vi "OP_Print_TPS_cluster_20170928.vi"() -> ()   [LabVIEW 2013]
uses:
  <vilib>/addons/database/Connection.llb/DB Tools Open Connec (Path).vi
  <vilib>/addons/database/Connection.llb/Conn Execute.vi
  <vilib>/addons/database/Recordset.llb/Rec Fetch Recordset Data (R).vi
  <vilib>/addons/database/Recordset.llb/Rec Destroy - Connection.vi
  <userlib>/caLab/Private/Get_PV-1D.vi
  <userlib>/caLab/Private/Get_PV.vi
  <vilib>/addons/database/NI_Database_API.lvlib
panel:
  in  "Refresh Button":bool
  in  "last ? Hrs":dbl=12.0 min=1.0 max=24.0 step=1.0
  out "error out 2":errorcluster
  out "x = y?":bool
  out "NOW time":string="21:22:35"
  out "NOW date":string="2017/09/13"
  in  "Save Button":bool
  out "error out 3":errorcluster
  in  "stop":bool
  out "time kickeron":string="21:11:02"
  out "date kickeron":string="2017/09/13"
  out "Cluster":T1={"SR Fill Pattern"=array[864 elements], "Beam Current(mA"=301.29559, "Beam Lifetime(min)"=467.3623843429031, "Beamsize X(um)"=61.81771808059018, "Beamsize Y(um)"=34.43346871436747, "Tune X(from BPM)"=0.0, "Tune Y(from BPM)"=0.0, "Mode"="Top-Up", "NuX(from BBF) "=0.15280663925802224, "NuY(from BBF)"=0.22496346361412184, "IU22-23gap(R)"=7.0, "IU22-05gap(R)"=7.28, "IU22-05M"=TRUE, "IU22A-09gap(R)"=8.058, "IU22A-09M"=TRUE, "IU22B-09gap(R)"=40.001, "IU22B-09M"=FALSE, "IUT22-21gap(R)"=7.0, "IUT22-21M"=TRUE, "IU22-23M"=TRUE, "IU22A-25gap(R)"=7.0, "IU22A-25M"=TRUE, "IU22B-25gap(R)"=40.0, "IU22B-25M"=FALSE, "EPU48A-41gap(R)"=65.0, "EPU48A-41gM"=FALSE, "EPU48B-41gap(R)"=44.99995, "EPU48B-41gM"=TRUE, "EPU46-45gap(R)"=65.00120000000001, "EPU46-45gM"=FALSE, "EPU48A-41phase(R)"=0.0009500000000000001, "EPU48B-41phase(R)"=0.0, "EPU46-45phase(R)"=0.0, "Grid volt.(V)(S)"=33.0, "Gun mode"="MBM", "Mod.3 HV(kV)(S)"=35.519999999999996, "SR"="SR_DMB_2017_0910_1700LOCO.data", "BR"="Booster_JT_2017_0714_1140.data", "Linac"="Linac_2017_0413_1015.data", "LTB"="LTB_JT_2017_0828_1050.data", "BTS"="BTS_2017_0911_0610.data", "RF2 remote"=TRUE, "RF2 OP mode"=TRUE, "RF2 phase.(S)"=-36.2, "RF Freq.(s)"=499655122.5507494, "RF2 gap volt.(S)"=1400.0, "RF3 remote"=TRUE, "RF3 OP mode"=TRUE, "RF3 phase.(S)"=9.000000000000004, "RF3 gap volt.(S)"=1400.0, "BBF V"=TRUE, "BBF H"=TRUE, "BR ext. kicker1(kV)"=17.666, "BR ext. kicker2(kV)"=17.666, "BR ext. sep.1(V)"=322.14, "BR ext. sep.2(V)"=441.1, "BR inj. sep.(V)"=104.95, "BR inj. kicker(kV)"=12.131749999999993, "SR kicker4(kV)"=8.133, "SR kicker3(kV)"=7.798, "SR kicker2(kV)"=8.259, "SR kicker1(kV)"=8.2, "SR inj. sep.2(V)"=397.2, "SR inj. sep.1(V)"=398.04, "Bucket Start"=100.0, "Bucket Last"=600.0, "Bucket Step"=10.0, "Orbit ILK(P)"=TRUE, "IU22-05 Hutch Enable"=TRUE, "IU22A-09M Hutch Enable"=TRUE, "IUT22-21M Hutch Enable"=TRUE, "IU22-23M Hutch Enable"=TRUE, "IU22A-25M Hutch Enable"=TRUE, "EPU48A-41M Hutch Enable"=FALSE, "EPU46-45M Hutch Enable"=FALSE, "EPU46-45 FE Enable"=TRUE, "EPU48A-41 FE Enable"=TRUE, "IU22A-25 FE Enable"=TRUE, "IU22-23 FE Enable"=TRUE, "IUT22-21 FE Enable"=TRUE, "IU22A-09 FE Enable"=TRUE, "IU22-05 FE Enable"=TRUE, "EPU48A-41pM"=FALSE, "EPU48B-41pM"=TRUE, "EPU46-45pM"=FALSE, "Gun volt.(V)(S)"=23.5, "Width count"=30.0, "2ns step"=0.0, "10ps delay"=150.0, "phase shifter"=130.0021, "Taper"=1.0899999999999999, "05XBPMX 1"=-12.071, "09XBPMX 1"=236.232, "21XBPMX 1"=109.949, "23XBPMX 1"=-54.123000000000005, "25XBPMX 1"=836.426, "41XBPMX 1"=-393.619, "45XBPMX 1"=-542.557, "05XBPMY 1"=49.623, "09XBPMY 1"=-49.685, "21XBPMY 1"=1810.249, "23XBPMY 1"=8.221, "25XBPMY 1"=-161.43800000000002, "41XBPMY 1"=188.45000000000002, "45XBPMY 1"=-785.827, "FOFB H"="On", "FOFB V"="On", "time string"="21:22:35", "date"="2017/09/13", "date (last kicker ON)"="2017/09/13", "time string (last kicker ON)"="21:11:02", "BPMX Graph"={[1, 2, 3, 4, 5, 6, 7, 8, 9, 10, 11, 12, 13, 14, 15, 16, 17, 18, 19, 20, 21, 22, 23, 24, 25, 26, 27, 28, 29, 30, 31, 32, 33, 34, 35, 36, 37, 38, 39, 40, 41, 42, 43, 44, 45, 46, 47, 48, 49, 50, 51, 52, 53, 54, 55, 56, 57, 58, 59, 60, 61, 62, 63, 64, 65, 66, 67, 68, 69, 70, 71, 72, 73, 74, 75, 76, 77, 78, 79, 80, 81, 82, 83, 84, 85, 86, 87, 88, 89, 90, 91, 92, 93, 94, 95, 96, 97, 98, 99, 100, 101, 102, 103, 104, 105, 106, 107, 108, 109, 110, 111, 112, 113, 114, 115, 116, 117, 118, 119, 120, 121, 122, 123, 124, 125, 126, 127, 128, 129, 130, 131, 132, 133, 134, 135, 136, 137, 138, 139, 140, 141, 142, 143, 144, 145, 146, 147, 148, 149, 150, 151, 152, 153, 154, 155, 156, 157, 158, 159, 160, 161, 162, 163, 164, 165, 166, 167, 168, 169, 170, 171, 172, 173, 174], "1rst Value (number)"=[-57.953, -16.830000000000002, -69.81400000000001, 33.217, 55.747, -102.116, 112.23700000000001, -53.109, -8.106, -108.797, 42.098, -26.618000000000002, 23.191, -14.290000000000001, -1.155, -135.518, -122.34, 81.94200000000001, -31.955000000000002, -107.23100000000001, 144.648, -41.501, -20.927, -71.483, 72.117, 174.239, 163.291, 218.172, -123.111, -19.648, 721.419, 453.44, -205.66400000000002, 29.594, 134.439, -81.831, 78.56700000000001, 81.661, 6.593, -174.97, 3.722, 159.74, -88.646, 74.924, 15.269, -34.265, -113.105, -24.846, 66.414, -131.589, 93.44500000000001, 99.491, -12.985, -180.05100000000002, 131.165, 37.079, -154.526, 160.38400000000001, 49.599000000000004, 24.96, -73.793, 85.367, 37.467, -10.198, 89.935, -39.093, 45.050000000000004, -60.443, 91.7, -89.60600000000001, -338.463, -13.786, -319.98900000000003, -247.719, -134.31, 117.925, -10.984, -69.336, 71.378, -119.991, 35.43, -76.868, 56.546, -1.875, -582.236, -130.956, -298.747, -39.141, 76.82900000000001, 82.033, -47.447, 68.075, 11.526, -161.376, 200.095, -3.3000000000000003, -170.391, -174.619, -59.896, 50.463, -167.593, 164.144, 6.708, -52.142, -152.178, 67.056, 8.861, -173.928, 197.31, 48.799, -71.952, -62.230000000000004, -4.128, 137.421, -127.104, 79.596, 56.283, -67.373, -122.31400000000001, 36.139, 42.783, -82.897, 55.373000000000005, 14.632, -53.128, -78.393, 32.919000000000004, -27.649, -194.787, 148.28300000000002, 205.038, -156.17600000000002, -87.652, -24.492, 101.044, -122.638, 98.552, 5.809, 62.325, -64.294, 38.297000000000004, 46.068, 274.628, 436.098, -130.642, -298.747, 133.037, 11.423, -153.334, 114.726, 76.023, -90.009, 92.394, 59.627, -74.368, -118.376, 43.591, 66.153, -129.306, 168.713, 4.539, -35.064, -130.217, 42.444, 59.192, -125.98400000000001, 147.53, 66.584, -28.801000000000002, -176.53, 75.164, 77.199, -57.284, -9.878]}, "BPMY Graph"={[1, 2, 3, 4, 5, 6, 7, 8, 9, 10, 11, 12, 13, 14, 15, 16, 17, 18, 19, 20, 21, 22, 23, 24, 25, 26, 27, 28, 29, 30, 31, 32, 33, 34, 35, 36, 37, 38, 39, 40, 41, 42, 43, 44, 45, 46, 47, 48, 49, 50, 51, 52, 53, 54, 55, 56, 57, 58, 59, 60, 61, 62, 63, 64, 65, 66, 67, 68, 69, 70, 71, 72, 73, 74, 75, 76, 77, 78, 79, 80, 81, 82, 83, 84, 85, 86, 87, 88, 89, 90, 91, 92, 93, 94, 95, 96, 97, 98, 99, 100, 101, 102, 103, 104, 105, 106, 107, 108, 109, 110, 111, 112, 113, 114, 115, 116, 117, 118, 119, 120, 121, 122, 123, 124, 125, 126, 127, 128, 129, 130, 131, 132, 133, 134, 135, 136, 137, 138, 139, 140, 141, 142, 143, 144, 145, 146, 147, 148, 149, 150, 151, 152, 153, 154, 155, 156, 157, 158, 159, 160, 161, 162, 163, 164, 165, 166, 167, 168, 169, 170, 171, 172, 173, 174], "1rst Value (number)"=[-151.316, -17.054000000000002, -19.178, 120.799, -59.688, 21.818, 7.809, -29.198, 24.311, 16.134, -40.005, -27.325, 53.925000000000004, 3.1670000000000003, -9.254, 61.293, -34.105000000000004, 94.741, -29.063, -23.54, 22.793, 14.087, -38.574, 36.56, -99.245, -0.044, 48.661, 33.093, -212.454, -68.398, 390.704, 121.525, -58.935, -19.379, 2.579, -18.495, 19.617, -37.129, 48.386, 12.363, -36.386, 3.988, 67.735, -11.383000000000001, 4.172, -13.203, 10.164, -0.589, -22.969, 30.752, -38.915, 41.105000000000004, -21.456, -4.901, 29.631, -9.992, -32.032000000000004, 12.132, -68.125, 97.674, -58.86, 66.602, -68.949, 58.512, -42.012, 22.742, -15.959, 12.297, 5.471, -82.755, 65.11, 15.540000000000001, -166.881, -18.198, 7.187, -10.503, 30.153000000000002, -70.941, -3.086, 7.163, -7.828, -18.855, 26.188, -7.574, 38.271, 0.135, -13.549, 40.546, 139.87800000000001, 4.58, -2.962, -6.871, 5.808, 0.435, 13.713000000000001, -7.65, -7.087, -2.88, 14.262, -32.895, 32.566, -5.7620000000000005, -44.698, 76.731, -22.138, 22.336000000000002, -6.075, -10.424, 12.001, -9.495000000000001, 18.714, -1.697, 7.412, -43.832, 47.095, -41.426, 2.965, 43.068, 29.560000000000002, -31.904, 28.699, -0.466, -7.138, -5.288, -15.559000000000001, 34.502, -45.603, -18.644000000000002, -3.043, -37.238, -6.869, -15.336, -4.0600000000000005, 13.134, -43.802, 53.087, -14.268, -32.236000000000004, 35.516, -16.788, 25.02, -56.714, 59.035000000000004, 117.801, 64.776, -29.192, -39.944, 137.099, -65.81700000000001, 24.237000000000002, -41.801, 16.21, 15.972, -22.743000000000002, 31.377, 18.596, 7.515000000000001, -19.796, 10.161, 1.0070000000000001, -7.114, -12.046, -4.223, 21.048000000000002, -8.239, -20.592, -8.097, 90.321, -136.733, 37.556, 84.604, -63.991, 30.307000000000002, 1.127]}, "Radio Buttons 2"=enum."absolute", "09XBPMX 2"="-47.22", "09XBPMY 2"="-3.76", "05XBPMY 2"="-491.14", "05XBPMX 2"="-472.70", "21XBPMY 2"=" closed", "21XBPMX 2"=" PAB ", "23XBPMY 2"="188.03", "23XBPMX 2"="-8.61", "25XBPMY 2"="5165.53", "25XBPMX 2"="2146.38", "41XBPMY 2"=" closed", "41XBPMX 2"=" Hutch ", "45XBPMX 2"=" Hutch ", "45XBPMY 2"=" closed", "05 mode"="Follow", "09A mode"="Follow", "09B mode"="Follow", "21 mode"="Follow", "23 mode"="Follow", "25A mode"="Follow", "25B mode"="Follow", "41A mode"="Follow", "41B mode"="Follow", "46 mode"="Follow", "BeamCurrent History"={"BPM NO.  1_172"=array[4320 elements], array[4320 elements]}, "SR Beam Current in            hours"=12.0} {"SR Beam Current in            hours" min=1.0 max=24.0 step=1.0 format="%#_2f"; "45XBPMY 1" format="%#.2f"; "41XBPMY 1" format="%#.2f"; "25XBPMY 1" format="%#.2f"; "23XBPMY 1" format="%#.2f"; "21XBPMY 1" format="%#.2f"; "09XBPMY 1" format="%#.2f"; "05XBPMY 1" format="%#.2f"; "45XBPMX 1" format="%#.2f"; "41XBPMX 1" format="%#.2f"; "25XBPMX 1" format="%#.2f"; "23XBPMX 1" format="%#.2f"; "21XBPMX 1" format="%#.2f"; "09XBPMX 1" format="%#.2f"; "05XBPMX 1" format="%#.2f"; "Taper" format="%#.4f"; "phase shifter" format="%#.3f"; "10ps delay" format="%#.1f"; "2ns step" format="%#.1f"; "Width count" format="%#.1f"; "Gun volt.(V)(S)" format="%#.1f"; "Bucket Step" format="%#.2f"; "Bucket Last" format="%#.2f"; "Bucket Start" format="%#.2f"; "BR ext. kicker1(kV)" format="%#.2f"; "BR ext. kicker2(kV)" format="%#.2f"; "BR ext. sep.1(V)" format="%#.2f"; "BR ext. sep.2(V)" format="%#.2f"; "BR inj. sep.(V)" format="%#.3f"; "BR inj. kicker(kV)" format="%#.3f"; "SR kicker4(kV)" format="%#.2f"; "SR kicker3(kV)" format="%#.2f"; "SR kicker2(kV)" format="%#.2f"; "SR kicker1(kV)" format="%#.2f"; "SR inj. sep.2(V)" format="%#.2f"; "SR inj. sep.1(V)" format="%#.2f"; "RF3 gap volt.(S)" format="%#.0f"; "RF3 phase.(S)" format="%#.1f"; "RF2 gap volt.(S)" format="%#.0f"; "RF Freq.(s)" format="%#.1f"; "RF2 phase.(S)" format="%#.1f"; "Mod.3 HV(kV)(S)" format="%#.3f"; "Grid volt.(V)(S)" format="%#.1f"; "EPU46-45phase(R)" format="%#.4f"; "EPU48B-41phase(R)" format="%#.4f"; "EPU48A-41phase(R)" format="%#.4f"; "EPU46-45gap(R)" format="%#.4f"; "EPU48B-41gap(R)" format="%#.4f"; "EPU48A-41gap(R)" format="%#.4f"; "IU22B-25gap(R)" format="%#.4f"; "IU22A-25gap(R)" format="%#.4f"; "IUT22-21gap(R)" format="%#.4f"; "IU22B-09gap(R)" format="%#.4f"; "IU22A-09gap(R)" format="%#.4f"; "IU22-05gap(R)" format="%#.4f"; "IU22-23gap(R)" format="%#.4f"; "NuY(from BBF)" format="%#.4f"; "NuX(from BBF)" format="%#.4f"; "Tune Y(from BPM)" format="%#.4f"; "Tune X(from BPM)" format="%#.4f"; "Beamsize Y(um)" format="%#.2f"; "Beamsize X(um)" format="%#.2f"; "Beam Lifetime(min)" format="%#.3f"; "Beam Current(mA" format="%#.3f"}
  out "date (last Gun ON)":string="2016/08/29"
  out "time string (last Gun ON)":string="23:28:50"
  out "Value Array (number) 7":dbl[](array[numeric])=[-12.071, 49.623, 236.232, -49.685, 109.949, 1810.249, -54.123000000000005, 8.221, 836.426, -161.43800000000002, -393.619, 188.45000000000002, -542.557, -785.827, -472.696, -491.142, -47.215, -3.761, 16.193, -29.476, -8.605, 188.026, 2146.382, 5165.525000000001, -28.331, 10.717, 132.828, -84.862]
  out "Value Array (number) 6":dbl[](array[numeric])=[7.28, 8.058, 40.001, 7.0, 7.0, 7.0, 40.0, 65.0, 0.0009500000000000001, 44.99995, 0.0, 65.00120000000001, 0.0, -1.0899999999999999, 130.0021]
  out "1rst Value (string) 2":string[](array[string])=["MBM", "33", "23.5", "350", "35.52", "22485", "22485", "62", "30", "0", "0", "200", "150"]
  out "Value Array (number) 5":dbl[](array[numeric])=[499654641.19275105, 1.0, 0.0, 1335.005102558433, 1400.0, -56.1, 1.0, 0.0, 1362.1066276040413, 1400.0, 160.0]
  out "1rst Value (string)":string[](array[string])=["Linac_2017_0413_1015.data", "LTB_JT_2017_0828_1050.data", "Booster_JT_2017_0714_1140.data", "BTS_2017_0911_0610.data", "SR_DMB_2017_0910_1700LOCO.data"]
  out "Value Array (number) 4":dbl[](array[numeric])=[499655122.5507494, 1.0, 0.0, 1326.2153542928932, 1400.0, -36.2, 1.0, 0.0, 1398.366426317367, 1400.0, 9.000000000000004]
  out "Value Array (number) 3":dbl[](array[numeric])=[0.0, 33.0, 23.5, 350.0, 35.519999999999996, 22485.0, 22485.0, 62.0, 30.0, 0.0, 0.0, 200.0, 150.0]
  out "Value Array (number) 2":dbl[](array[numeric])=[104.95, 12.131749999999993, 17.666, 17.666, 322.14, 441.1, 398.04, 397.2, 8.2, 8.259, 7.798, 8.133]
  out "Value Array (number)":dbl[](array[numeric])=[1.0, 301.29559, 467.3623843429031, 51.42904998385207, 28.64681257434898, 0.1761252446183953, 0.12524461839530332, 88.36853790283203, 130.0970458984375, 100.0, 600.0, 10.0]
  out "Orbit ILK(A)":bool
  out "Orbit INT. Ang Active":bool
  out "Orbit INT.Ang. On":bool
  out "Orbit INT. Pos Active":bool
  out "Orbit INT.Pos. On":bool
  out "SBM volt.(S)":dbl=350.0 format="%#.1f"
  out "MBM volt.(S)":dbl=23.5 format="%#.1f"
  in  "Copy Button":bool
  in  "Print Button":bool
  in  "Help Button":bool
  in  "Refresh Button":bool
  in  "Open Button":bool
  out "Gun WCM":dbl[](graph)
  out "BR Fill Pattern":dbl[](graph)
  # "TPS OP Handover Information"
  # "Others"
  # "Time："
  # "Valve  Status"
  # "follow"
  # "SM Status"
  # "歷史電流圖\ntrip次數?\n輻射劑量?\n平均氣壓\n目前最高累計劑量\n最近一次觸發時BR電流及WCM數值"
  # "TPS Operational Handover Information v1.4.1"
  # "SR Status"
  # "Feedback"
  # "Pulse Mag"
  # "LINAC"
  # "x8(ns)"
  # "x2(ns)"
  # "x0.01(ns)"
  # "RF Status"
  # "Hz"
  # "(kV)"
  # "(kV)"
  # "Changeliang@LOP.NSRRC"
  # "SR Fill Pattern"
  # "Lattice Files in using"
  # "ID &Beamline (R)"
  # "mode"
  # "Gap\nmm"
  # "Motor"
  # "Phase"
  # "FE/Hutch"
  # "phase\nshifter"
  # "Taper\n(enc)"
  # "XBPM1X\num"
  # "XBPM1Y\num"
  # "XBPM2X\num"
  # "XBPM2Y\num"
  # "05"
  # "09"
  # "21"
  # "23"
  # "25"
  # "41"
  # "45"
  # "SR Orbit"
  # "BPMX"
  # "BPMY"
  # "SR Beam Current History"
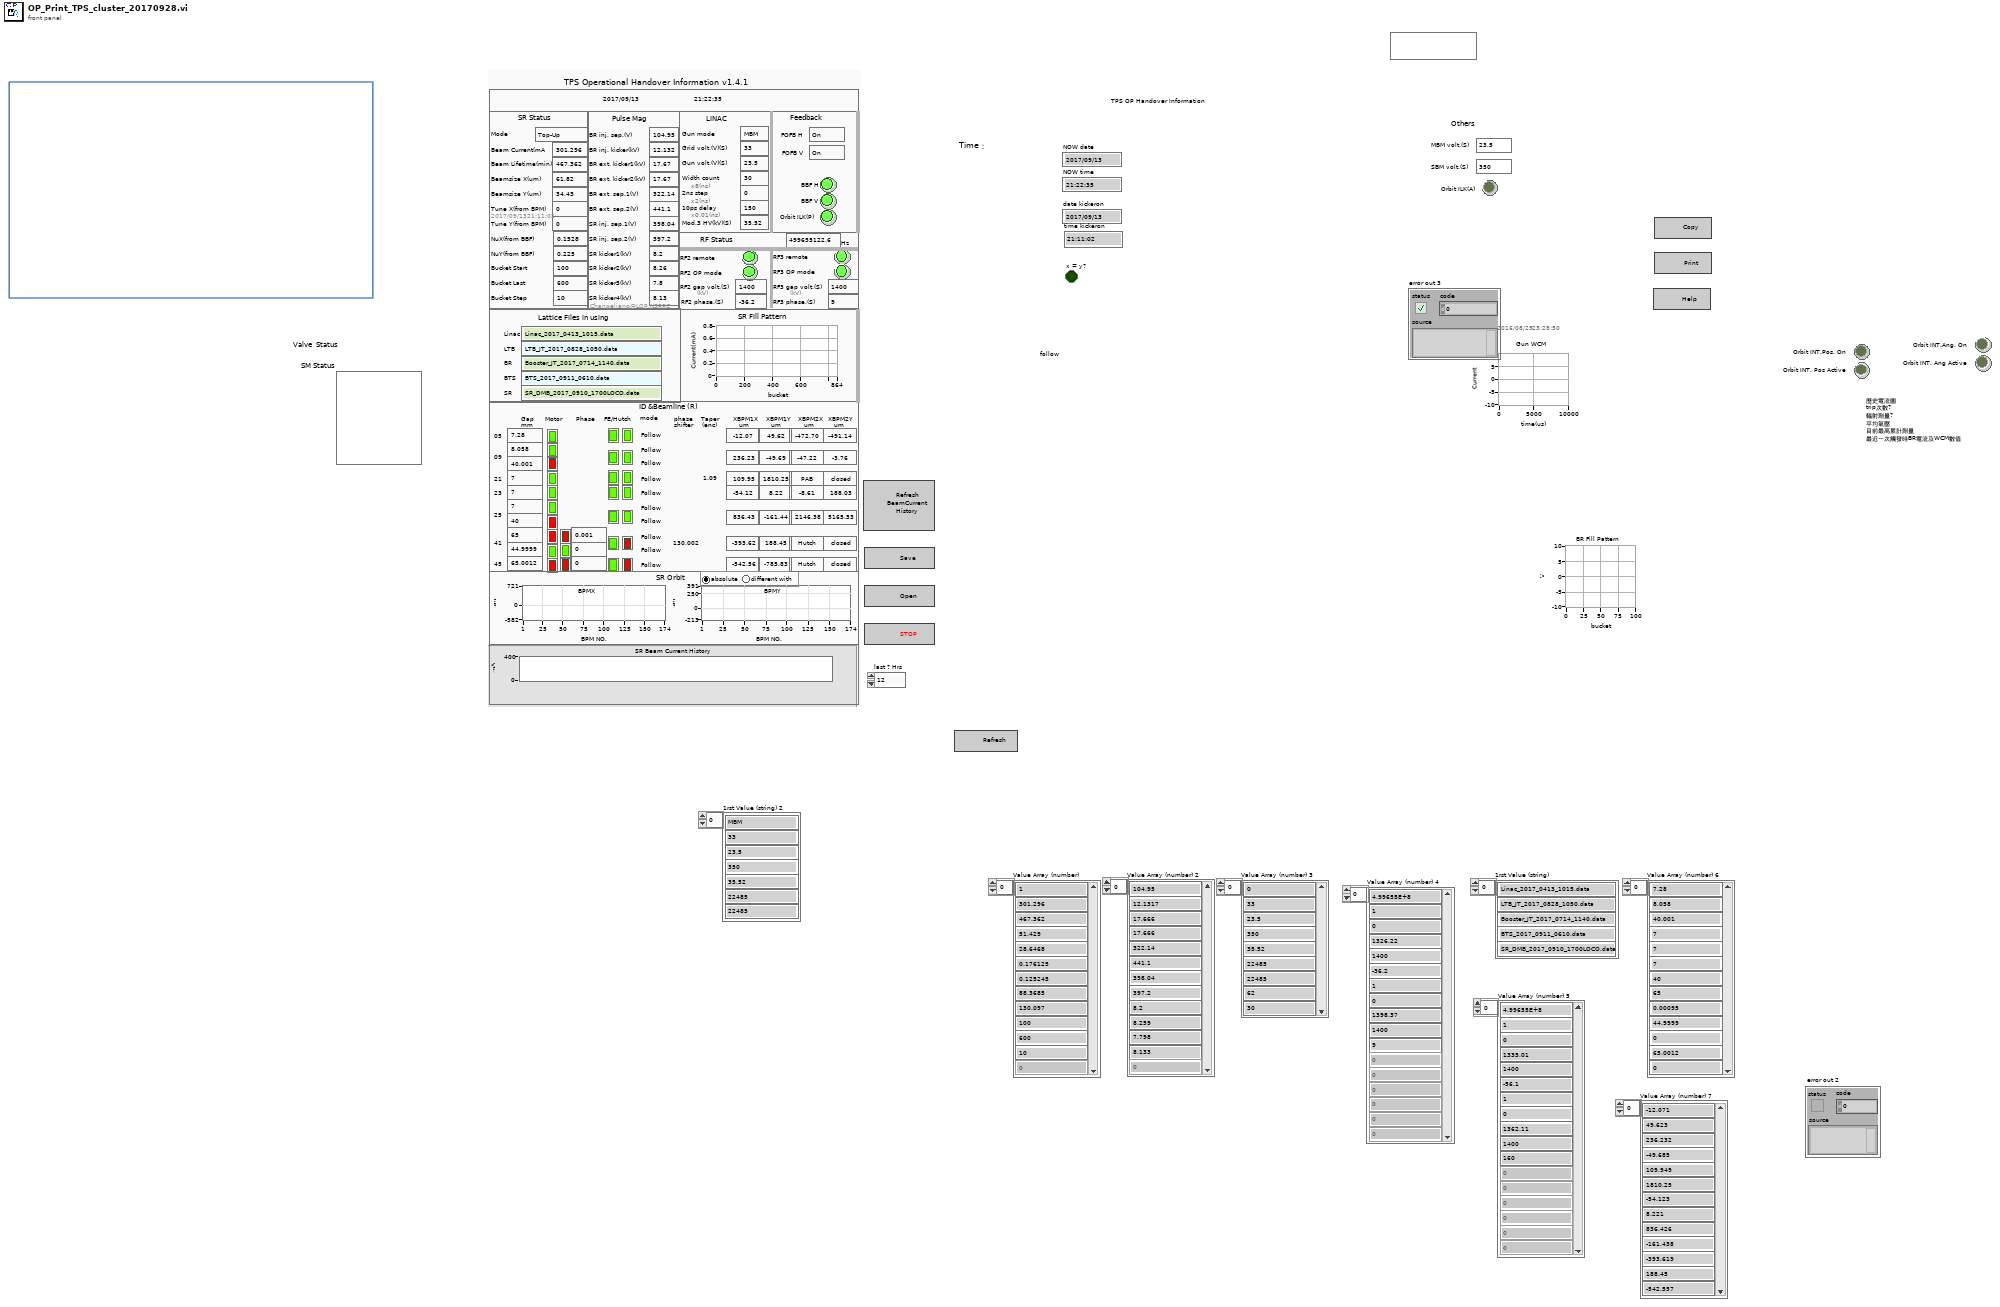
[diagram p1: front panel]
types:
  T1 = cluster{"SR Fill Pattern":dbl[], "Beam Current(mA":dbl, "Beam Lifetime(min)":dbl, "Beamsize X(um)":dbl, "Beamsize Y(um)":dbl, "Tune X(from BPM)":dbl, "Tune Y(from BPM)":dbl, "Mode":string, "NuX(from BBF) ":dbl, "NuY(from BBF)":dbl, "IU22-23gap(R)":dbl, "IU22-05gap(R)":dbl, "IU22-05M":bool, "IU22A-09gap(R)":dbl, "IU22A-09M":bool, "IU22B-09gap(R)":dbl, "IU22B-09M":bool, "IUT22-21gap(R)":dbl, "IUT22-21M":bool, "IU22-23M":bool, "IU22A-25gap(R)":dbl, "IU22A-25M":bool, "IU22B-25gap(R)":dbl, "IU22B-25M":bool, "EPU48A-41gap(R)":dbl, "EPU48A-41gM":bool, "EPU48B-41gap(R)":dbl, "EPU48B-41gM":bool, "EPU46-45gap(R)":dbl, "EPU46-45gM":bool, "EPU48A-41phase(R)":dbl, "EPU48B-41phase(R)":dbl, "EPU46-45phase(R)":dbl, "Grid volt.(V)(S)":dbl, "Gun mode":string, "Mod.3 HV(kV)(S)":dbl, "SR":string, "BR":string, "Linac":string, "LTB":string, "BTS":string, "RF2 remote":bool, "RF2 OP mode":bool, "RF2 phase.(S)":dbl, "RF Freq.(s)":dbl, "RF2 gap volt.(S)":dbl, "RF3 remote":bool, "RF3 OP mode":bool, "RF3 phase.(S)":dbl, "RF3 gap volt.(S)":dbl, "BBF V":bool, "BBF H":bool, "BR ext. kicker1(kV)":dbl, "BR ext. kicker2(kV)":dbl, "BR ext. sep.1(V)":dbl, "BR ext. sep.2(V)":dbl, "BR inj. sep.(V)":dbl, "BR inj. kicker(kV)":dbl, "SR kicker4(kV)":dbl, "SR kicker3(kV)":dbl, "SR kicker2(kV)":dbl, "SR kicker1(kV)":dbl, "SR inj. sep.2(V)":dbl, "SR inj. sep.1(V)":dbl, "Bucket Start":dbl, "Bucket Last":dbl, "Bucket Step":dbl, "Orbit ILK(P)":bool, "IU22-05 Hutch Enable":bool, "IU22A-09M Hutch Enable":bool, "IUT22-21M Hutch Enable":bool, "IU22-23M Hutch Enable":bool, "IU22A-25M Hutch Enable":bool, "EPU48A-41M Hutch Enable":bool, "EPU46-45M Hutch Enable":bool, "EPU46-45 FE Enable":bool, "EPU48A-41 FE Enable":bool, "IU22A-25 FE Enable":bool, "IU22-23 FE Enable":bool, "IUT22-21 FE Enable":bool, "IU22A-09 FE Enable":bool, "IU22-05 FE Enable":bool, "EPU48A-41pM":bool, "EPU48B-41pM":bool, "EPU46-45pM":bool, "Gun volt.(V)(S)":dbl, "Width count":dbl, "2ns step":dbl, "10ps delay":dbl, "phase shifter":dbl, "Taper":dbl, "05XBPMX 1":dbl, "09XBPMX 1":dbl, "21XBPMX 1":dbl, "23XBPMX 1":dbl, "25XBPMX 1":dbl, "41XBPMX 1":dbl, "45XBPMX 1":dbl, "05XBPMY 1":dbl, "09XBPMY 1":dbl, "21XBPMY 1":dbl, "23XBPMY 1":dbl, "25XBPMY 1":dbl, "41XBPMY 1":dbl, "45XBPMY 1":dbl, "FOFB H":string, "FOFB V":string, "time string":string, "date":string, "date (last kicker ON)":string, "time string (last kicker ON)":string, "BPMX Graph":cluster{i32[], "1rst Value (number)":dbl[]}, "BPMY Graph":cluster{i32[], "1rst Value (number)":dbl[]}, "Radio Buttons 2":enum32{"absolute", "different with"}, "09XBPMX 2":string, "09XBPMY 2":string, "05XBPMY 2":string, "05XBPMX 2":string, "21XBPMY 2":string, "21XBPMX 2":string, "23XBPMY 2":string, "23XBPMX 2":string, "25XBPMY 2":string, "25XBPMX 2":string, "41XBPMY 2":string, "41XBPMX 2":string, "45XBPMX 2":string, "45XBPMY 2":string, "05 mode":string, "09A mode":string, "09B mode":string, "21 mode":string, "23 mode":string, "25A mode":string, "25B mode":string, "41A mode":string, "41B mode":string, "46 mode":string, "BeamCurrent History":cluster{"BPM NO.  1_172":dbl[], dbl[]}, "SR Beam Current in            hours":dbl}
  T2 = typedef "NI_Database_API.lvlib/Conn ObjectReference.ctl" = refnum<k1>
  T3 = typedef "NI_Database_API.lvlib/Rec ObjectReference.ctl" = refnum<k1>
  T4 = cluster{"SR Fill Pattern":dbl[], "Beam Current(mA":dbl, "Beam Lifetime(min)":dbl, "Beamsize X(um)":dbl, "Beamsize Y(um)":dbl, "Tune X(from BPM)":dbl, "Tune Y(from BPM)":dbl, "Mode":string, "NuX(from BBF) ":dbl, "NuY(from BBF)":dbl, "IU22-23gap(R)":dbl, "IU22-05gap(R)":dbl, "IU22-05M":bool, "IU22A-09gap(R)":dbl, "IU22A-09M":bool, "IU22B-09gap(R)":dbl, "IU22B-09M":bool, "IUT22-21gap(R)":dbl, "IUT22-21M":bool, "IU22-23M":bool, "IU22A-25gap(R)":dbl, "IU22A-25M":bool, "IU22B-25gap(R)":dbl, "IU22B-25M":bool, "EPU48A-41gap(R)":dbl, "EPU48A-41gM":bool, "EPU48B-41gap(R)":dbl, "EPU48B-41gM":bool, "EPU46-45gap(R)":dbl, "EPU46-45gM":bool, "EPU48A-41phase(R)":dbl, "EPU48B-41phase(R)":dbl, "EPU46-45phase(R)":dbl, "Grid volt.(V)(S)":dbl, "Gun mode":string, "Mod.3 HV(kV)(S)":dbl, "SR":string, "BR":string, "Linac":string, "LTB":string, "BTS":string, "RF2 remote":bool, "RF2 OP mode":bool, "RF2 phase.(S)":dbl, "RF Freq.(s)":dbl, "RF2 gap volt.(S)":dbl, "RF3 remote":bool, "RF3 OP mode":bool, "RF3 phase.(S)":dbl, "RF3 gap volt.(S)":dbl, "BBF V":bool, "BBF H":bool, "BR ext. kicker1(kV)":dbl, "BR ext. kicker2(kV)":dbl, "BR ext. sep.1(V)":dbl, "BR ext. sep.2(V)":dbl, "BR inj. sep.(V)":dbl, "BR inj. kicker(kV)":dbl, "SR kicker4(kV)":dbl, "SR kicker3(kV)":dbl, "SR kicker2(kV)":dbl, "SR kicker1(kV)":dbl, "SR inj. sep.2(V)":dbl, "SR inj. sep.1(V)":dbl, "Bucket Start":dbl, "Bucket Last":dbl, "Bucket Step":dbl, "Orbit ILK(P)":bool, "IU22-05 Hutch Enable":bool, "IU22A-09M Hutch Enable":bool, "IUT22-21M Hutch Enable":bool, "IU22-23M Hutch Enable":bool, "IU22A-25M Hutch Enable":bool, "EPU48A-41M Hutch Enable":bool, "EPU46-45M Hutch Enable":bool, "EPU46-45 FE Enable":bool, "EPU48A-41 FE Enable":bool, "IU22A-25 FE Enable":bool, "IU22-23 FE Enable":bool, "IUT22-21 FE Enable":bool, "IU22A-09 FE Enable":bool, "IU22-05 FE Enable":bool, "EPU48A-41pM":bool, "EPU48B-41pM":bool, "EPU46-45pM":bool, "Gun volt.(V)(S)":dbl, "Width count":dbl, "2ns step":dbl, "10ps delay":dbl, "phase shifter":dbl, "Taper":dbl, "05XBPMX 1":dbl, "09XBPMX 1":dbl, "21XBPMX 1":dbl, "23XBPMX 1":dbl, "25XBPMX 1":dbl, "41XBPMX 1":dbl, "45XBPMX 1":dbl, "05XBPMY 1":dbl, "09XBPMY 1":dbl, "21XBPMY 1":dbl, "23XBPMY 1":dbl, "25XBPMY 1":dbl, "41XBPMY 1":dbl, "45XBPMY 1":dbl, "FOFB H":string, "FOFB V":string, "time string":string, "date":string, "date (last kicker ON)":string, "time string (last kicker ON)":string, "BPMX Graph":cluster{i32[], "1rst Value (number)":dbl[]}, "BPMY Graph":cluster{i32[], "1rst Value (number)":dbl[]}, "Radio Buttons 2":enum32{"absolute", "different with"}, "09XBPMX 2":string, "09XBPMY 2":string, "05XBPMY 2":string, "05XBPMX 2":string, "21XBPMY 2":string, "21XBPMX 2":string, "23XBPMY 2":string, "23XBPMX 2":string, "25XBPMY 2":string, "25XBPMX 2":string, "41XBPMY 2":string, "41XBPMX 2":string, "45XBPMX 2":string, "45XBPMY 2":string, "05 mode":string, "09A mode":string, "09B mode":string, "21 mode":string, "23 mode":string, "25A mode":string, "25B mode":string, "41A mode":string, "41B mode":string, "46 mode":string, "BeamCurrent History":cluster{"BPM NO.  1_172":dbl[], dbl[]}, "SR Beam Current in Last           Hrs":dbl}
  T5 = typedef "imagedata.ctl" = cluster{"image type":i32, "image depth":i32, "image":u8[], "mask":u8[], "colors":u32[], "Rectangle":cluster{"left":i16, "top":i16, "right":i16, "bottom":i16}}
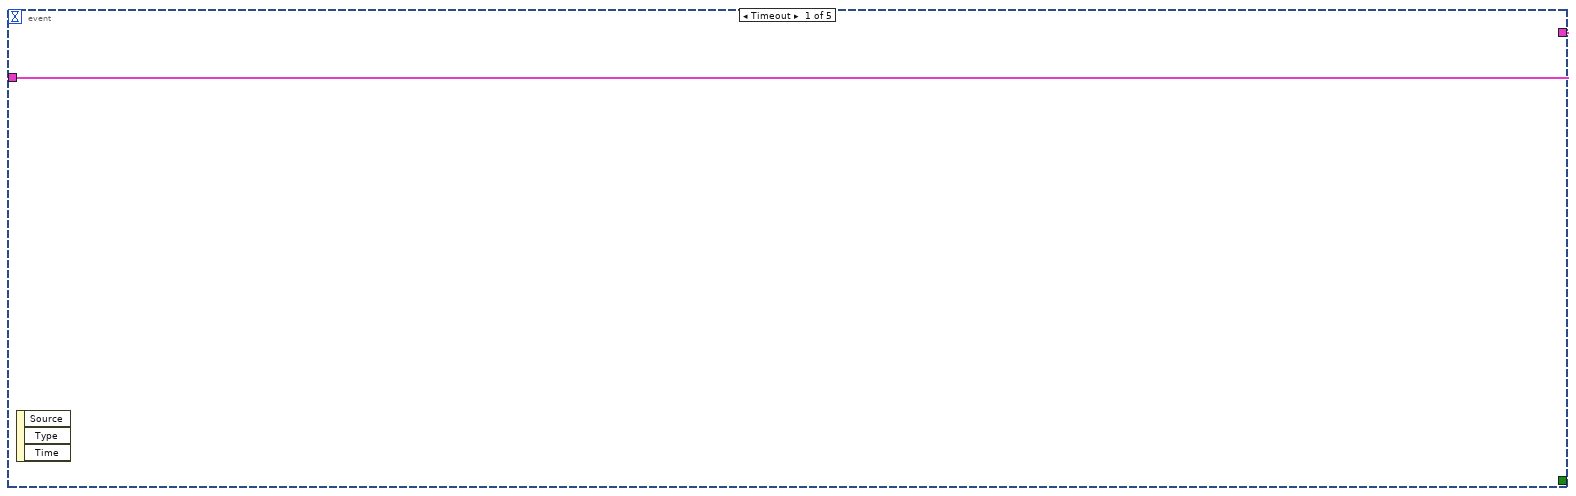
[diagram p4: hidden frame]
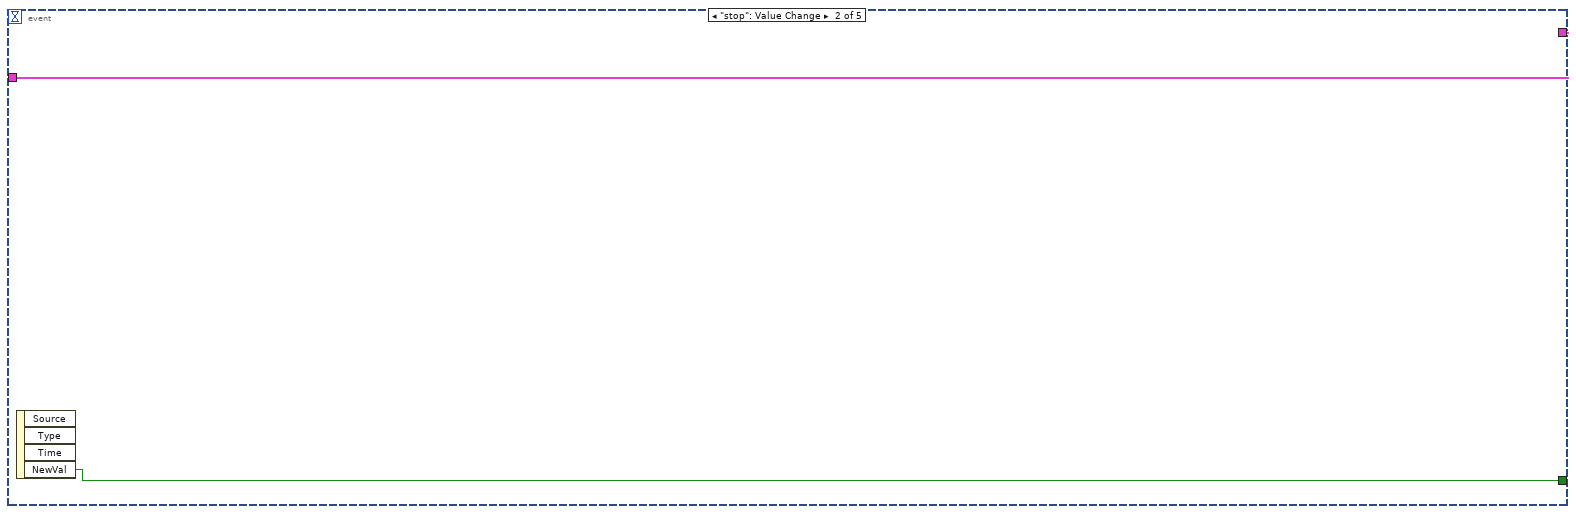
[diagram p5: hidden frame]
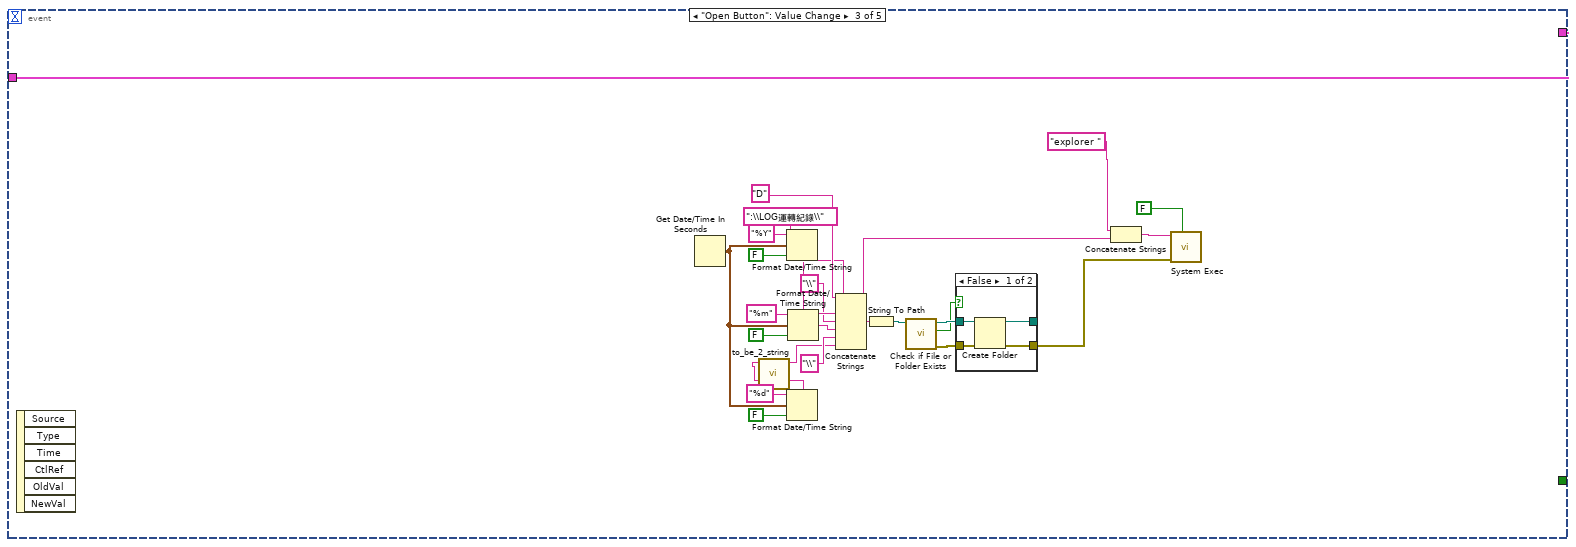
[diagram p6: hidden frame]
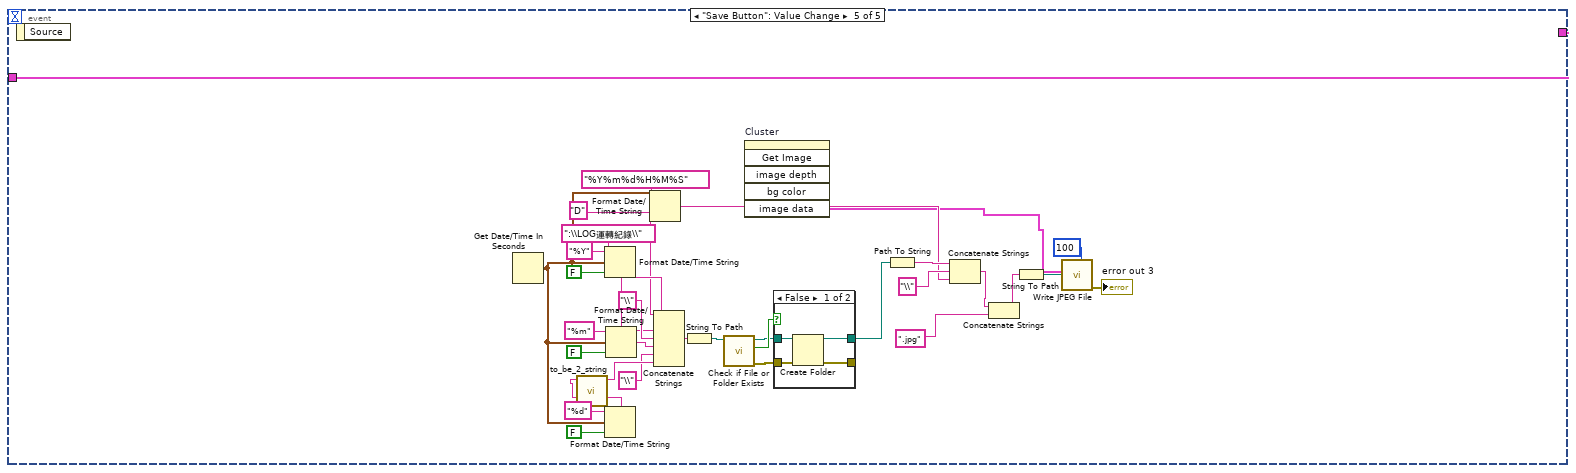
[diagram p8: hidden frame]
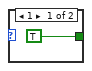
[diagram p10: hidden frame]
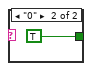
[diagram p13: hidden frame]
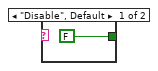
[diagram p14: hidden frame]
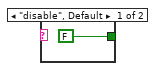
[diagram p15: hidden frame]
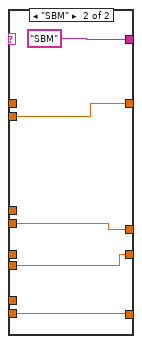
[diagram p16: hidden frame]
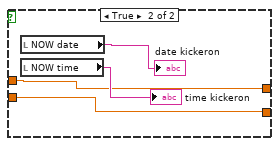
[diagram p17: hidden frame]
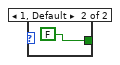
[diagram p18: hidden frame]
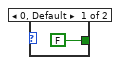
[diagram p19: hidden frame]
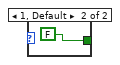
[diagram p20: hidden frame]
diagram:
  (unwired) string[] ["FE-DI-XBPM-051:SA:SA_X_MONITOR", "FE-DI-XBPM-051:SA:SA_Y_MONITOR", "FE-DI-XBPM-091:SA:SA_X_MONITOR", "FE-DI-XBPM-091:SA:SA_Y_MONITOR", "FE-DI-XBPM-211:SA:SA_X_MONITOR", "FE-DI-XBPM-211:SA:SA_Y_MONITOR", "FE-DI-XBPM-231:SA:SA_X_MONITOR", "FE-DI-XBPM-231:SA:SA_Y_MONITOR", "FE-DI-XBPM-251:SA:SA_X_MONITOR", "FE-DI-XBPM-251:SA:SA_Y_MONITOR", "FE-DI-XBPM-411:SA:SA_X_MONITOR", "FE-DI-XBPM-411:SA:SA_Y_MONITOR", "FE-DI-XBPM-451:SA:SA_X_MONITOR", "FE-DI-XBPM-451:SA:SA_Y_MONITOR"]
  (unwired) string[] ["LI-VA-VAL-01:STA:POS", "LI-VA-VAL-02:STA:POS", "LI-VA-VAL-03:STA:POS", "LI-VA-VAL-04:STA:POS", "LI-VA-VAL-05:STA:POS"]
  (unwired) string[] ["SR-DI-SOFB-H:getStatus", "SR-DI-SOFB-V:getStatus", "IGPF:TPSX:FBCTRL", "IGPF:TPSY:FBCTRL", "SR-DI-FOFB-H:getStatus", "SR-DI-FOFB-V:getStatus"]
  # "1.4.1\n將BeamCurrent 圖形的Y軸上下限\n改成取最大值的1.01倍，再無條件進位取整數\n最小值的0.99倍，再無條件捨去取整數"
  # "FE-DI-XBPM-051:SA:SA_Y_MONITOR"
  # "FE-DI-XBPM-051:SA:SA_X_MONITOR"
  # "TPS-SR-052:bpm4:ilk:enabled"
  # "0 為OPEN"
  # "VALVE(EPICS)"
  n1 = local read "last ? Hrs"() -> (w15:dbl)
  n2 = Multiply(x=3600.0 ("y"), y=w15) -> (x*y=w39:dbl)
  n3 = Get Date/Time In Seconds() -> (seconds since 1Jan1904=w3:timestamp)
  n4 = Subtract(x=w3, y=w39) -> (x-y=w2:timestamp)
  n5 = call "TimeToString.vi"("Time Stamp Control"=w3) -> ("result string"=w41:string)
  n6 = call "TimeToString.vi"("Time Stamp Control"=w2) -> ("result string"=w40:string)
  n7 = call <vilib>:"Application Directory.vi"() -> ("Application Directory"=w42:path)
  n8 = Build Path(base path=w42, name or relative path="DSN\\172-18-0-32.dsn") -> (appended path=w44:path)
  n9 = call-poly <vilib>:"DB Tools Open Connection.vi"("connection information"=w44) -> ("error out"=w33:errorcluster, "connection reference"=w32:T2)  [unwired: 7 in]
  n10 = Concatenate Strings("SELECT  float_val , smpl_time\nFROM sample \nwhere  channel_id = 104 and smpl_time between '" ("result string"), w40, "' ::timestamp and '" ("result string"), w41, "' ::timestamp" ("result string")) -> (w17:string)
  n11 = call-poly <vilib>:"DB Tools Execute Query.vi"("error in (no error)"=w33, "SQL query"=w17, "connection reference"=w32) -> ("error out"=w30:errorcluster, "recordset reference"=w31:T3)  [unwired: 5 in]
  n12 = call-poly <vilib>:"DB Tools Fetch Recordset Data.vi"("error in (no error)"=w30, "recordset reference"=w31) -> ("error out"=w28:errorcluster, "recordset data"=w25:variant[][], "recordset reference out"=w29:T3)  [unwired: 3 in]
  n13 = call-poly <vilib>:"DB Tools Free Object.vi"("error in (no error)"=w28, "recordset reference"=w29) -> ("error out"=w26:errorcluster, "connection reference"=w27:T2)  [unwired: 8 in]
  n14 = Variant To Data(type=string[][] [], Variant=w25) -> (data=w23:string[][])  [unwired: 1 in, 1 out]
  n15 = call <vilib>:"DB Tools Close Connection.vi"("error in (no error)"=w26, "connection reference"=w27) -> ()  [unwired: 5 in, 1 out]
  n16 = Transpose 2D Array(2D array=w23) -> (transposed array=w21:string[][])
  n17 = Index Array(array=w21, index (row) #1=0 ("index (row)"), index (row) #2=1 ("index (row)")) -> (element #1=w35:string[], element #2=w37:string[])  [unwired: 2 in]
  n18 = Fract/Exp String To Number(string=w35) -> (number=w4:dbl[])  [unwired: 3 in, 1 out]
  n19 = Array Max & Min(array=w4) -> (max value=w1:dbl, min value=w11:dbl)  [unwired: 2 out]
  n20 = for {
    tunnel: w37 -> [w48] mode=indexing
    tunnel: [w47] -> w36 mode=indexing
    n21 = Scan From String "Scan From String"(format string="%<%Y/%m/%d %p %I:%M:%S>T", input string=w48, initial scan location=u32 0, default 1=timestamp(-73814400 s since 1904-01-01)) -> (output 1=w51:timestamp)  [unwired: 1 in, 3 out]
    n22 = To Double Precision Float(number=w51) -> (double precision float=w47:dbl)
  }
  n23 = Multiply(x=w1, y=1.01) -> (x*y=w9:dbl)
  n24 = Multiply(x=w11, y=0.99) -> (x*y=w12:dbl)
  n25 = Round Toward +Infinity(x=w9) -> (ceil(x): smallest int >= x=w14:dbl)
  n26 = Round Toward -Infinity(1:w12) -> (0:w13:dbl)
  n27 = To Double Precision Float(number=w3) -> (double precision float=w6:dbl)
  n28 = To Double Precision Float(number=w2) -> (double precision float=w5:dbl)
  n29 = control-ref of="BeamCurrent History"() -> (w7:refnum<vi>)
  n30 = property on="Property Node" class="XYGraph (strict)"(reference=w7, "XScale.Maximum"=w6, "XScale.Minimum"=w5, "YScale.Maximum"=w14, "YScale.Minimum"=w13) -> ()  [unwired: 1 in, 2 out]
  n31 = Bundle(w36, w4) -> (w16:cluster{dbl[], dbl[]})  [unwired: 1 in]
  n32 = while {
    shift-right: [w193] -> _
    shift-left: _ -> [w191]
    shift-right: [w192] -> _
    shift-left: _ -> [w190]
    shift-right: [w53] -> _
    shift-left: w16 -> [w52]
    stop <- "stop" stop-if-true
    w80 = string[] ["SR-ID-IU22-05:setECMode", "SR-ID-IU22A-09:setECMode", "SR-ID-IU22B-09:setECMode", "SR-ID-IUT22-21:setECMode", "SR-ID-IU22-23:setECMode", "SR-ID-IU22A-25:setECMode", "SR-ID-IU22B-25:setECMode", "SR-ID-EPU48A-41:setECMode", "SR-ID-EPU48B-41:setECMode", "SR-ID-EPU46-45:setECMode"]  # ID_mode
    w166 = string[] ["FE-05-PAB:Open", "FE-05-MGV:Open", "FE-05-FCV:Open", "FE-09-PAB:Open", "FE-09-MGV:Open", "FE-09-FCV:Open", "FE-21-PAB:Open", "FE-21-MGV:Open", "FE-21-FCV:Open", "FE-23-PAB:Open", "FE-23-PAB:Open", "FE-23-FCV:Open", "FE-25-PAB:Open", "FE-25-MGV:Open", "FE-25-FCV:Open", "FE-41-PAB:Open", "FE-41-MGV:Open", "FE-41-FCV:Open", "FE-45-PAB:Open", "FE-45-MGV:Open", "FE-45-FCV:Open"]  # PAB_MGV_FCV enable
    (unwired) "LI-DI-WCM:getWfCh1"
    (unwired) "SR-DI-FP:CurrentBuffer"
    w313 = i32[] [1, 2, 3, 4, 5, 6, 7, 8, 9, 10, 11, 12, 13, 14, 15, 16, 17, 18, 19, 20, 21, 22, 23, 24, 25, 26, 27, 28, 29, 30, 31, 32, 33, 34, 35, 36, 37, 38, 39, 40, 41, 42, 43, 44, 45, 46, 47, 48, 49, 50, 51, 52, 53, 54, 55, 56, 57, 58, 59, 60, 61, 62, 63, 64, 65, 66, 67, 68, 69, 70, 71, 72, 73, 74, 75, 76, 77, 78, 79, 80, 81, 82, 83, 84, 85, 86, 87, 88, 89, 90, 91, 92, 93, 94, 95, 96, 97, 98, 99, 100, 101, 102, 103, 104, 105, 106, 107, 108, 109, 110, 111, 112, 113, 114, 115, 116, 117, 118, 119, 120, 121, 122, 123, 124, 125, 126, 127, 128, 129, 130, 131, 132, 133, 134, 135, 136, 137, 138, 139, 140, 141, 142, 143, 144, 145, 146, 147, 148, 149, 150, 151, 152, 153, 154, 155, 156, 157, 158, 159, 160, 161, 162, 163, 164, 165, 166, 167, 168, 169, 170, 171, 172, 173, 174] ("Array 4")
    w311 = 0.001
    w309 = string[] ["SR-DI-BPM-011:Y", "SR-DI-BPM-012:Y", "SR-DI-BPM-013:Y", "SR-DI-BPM-014:Y", "SR-DI-BPM-015:Y", "SR-DI-BPM-016:Y", "SR-DI-BPM-017:Y", "SR-DI-BPM-021:Y", "SR-DI-BPM-022:Y", "SR-DI-BPM-023:Y", "SR-DI-BPM-024:Y", "SR-DI-BPM-025:Y", "SR-DI-BPM-026:Y", "SR-DI-BPM-027:Y", "SR-DI-BPM-031:Y", "SR-DI-BPM-032:Y", "SR-DI-BPM-033:Y", "SR-DI-BPM-034:Y", "SR-DI-BPM-035:Y", "SR-DI-BPM-036:Y", "SR-DI-BPM-037:Y", "SR-DI-BPM-041:Y", "SR-DI-BPM-042:Y", "SR-DI-BPM-043:Y", "SR-DI-BPM-044:Y", "SR-DI-BPM-045:Y", "SR-DI-BPM-046:Y", "SR-DI-BPM-047:Y", "SR-DI-BPM-048:Y", "SR-DI-BPM-050:Y", "SR-DI-BPM-051:Y", "SR-DI-BPM-052:Y", "SR-DI-BPM-053:Y", "SR-DI-BPM-054:Y", "SR-DI-BPM-055:Y", "SR-DI-BPM-056:Y", "SR-DI-BPM-057:Y", "SR-DI-BPM-061:Y", "SR-DI-BPM-062:Y", "SR-DI-BPM-063:Y", "SR-DI-BPM-064:Y", "SR-DI-BPM-065:Y", "SR-DI-BPM-066:Y", "SR-DI-BPM-067:Y", "SR-DI-BPM-071:Y", "SR-DI-BPM-072:Y", "SR-DI-BPM-073:Y", "SR-DI-BPM-074:Y", "SR-DI-BPM-075:Y", "SR-DI-BPM-076:Y", "SR-DI-BPM-077:Y", "SR-DI-BPM-081:Y", "SR-DI-BPM-082:Y", "SR-DI-BPM-083:Y", "SR-DI-BPM-084:Y", "SR-DI-BPM-085:Y", "SR-DI-BPM-086:Y", "SR-DI-BPM-087:Y", "SR-DI-BPM-091:Y", "SR-DI-BPM-092:Y", "SR-DI-BPM-093:Y", "SR-DI-BPM-094:Y", "SR-DI-BPM-095:Y", "SR-DI-BPM-096:Y", "SR-DI-BPM-097:Y", "SR-DI-BPM-101:Y", "SR-DI-BPM-102:Y", "SR-DI-BPM-103:Y", "SR-DI-BPM-104:Y", "SR-DI-BPM-105:Y", "SR-DI-BPM-106:Y", "SR-DI-BPM-107:Y", "SR-DI-BPM-111:Y", "SR-DI-BPM-112:Y", "SR-DI-BPM-113:Y", "SR-DI-BPM-114:Y", "SR-DI-BPM-115:Y", "SR-DI-BPM-116:Y", "SR-DI-BPM-117:Y", "SR-DI-BPM-121:Y", "SR-DI-BPM-122:Y", "SR-DI-BPM-123:Y", "SR-DI-BPM-124:Y", "SR-DI-BPM-125:Y", "SR-DI-BPM-126:Y", "SR-DI-BPM-127:Y", "SR-DI-BPM-128:Y", "SR-DI-BPM-130:Y", "SR-DI-BPM-131:Y", "SR-DI-BPM-132:Y", "SR-DI-BPM-133:Y", "SR-DI-BPM-134:Y", "SR-DI-BPM-135:Y", "SR-DI-BPM-136:Y", "SR-DI-BPM-137:Y", "SR-DI-BPM-141:Y", "SR-DI-BPM-142:Y", "SR-DI-BPM-143:Y", "SR-DI-BPM-144:Y", "SR-DI-BPM-145:Y", "SR-DI-BPM-146:Y", "SR-DI-BPM-147:Y", "SR-DI-BPM-151:Y", "SR-DI-BPM-152:Y", "SR-DI-BPM-153:Y", "SR-DI-BPM-154:Y", "SR-DI-BPM-155:Y", "SR-DI-BPM-156:Y", "SR-DI-BPM-157:Y", "SR-DI-BPM-161:Y", "SR-DI-BPM-162:Y", "SR-DI-BPM-163:Y", "SR-DI-BPM-164:Y", "SR-DI-BPM-165:Y", "SR-DI-BPM-166:Y", "SR-DI-BPM-167:Y", "SR-DI-BPM-171:Y", "SR-DI-BPM-172:Y", "SR-DI-BPM-173:Y", "SR-DI-BPM-174:Y", "SR-DI-BPM-175:Y", "SR-DI-BPM-176:Y", "SR-DI-BPM-177:Y", "SR-DI-BPM-181:Y", "SR-DI-BPM-182:Y", "SR-DI-BPM-183:Y", "SR-DI-BPM-184:Y", "SR-DI-BPM-185:Y", "SR-DI-BPM-186:Y", "SR-DI-BPM-187:Y", "SR-DI-BPM-191:Y", "SR-DI-BPM-192:Y", "SR-DI-BPM-193:Y", "SR-DI-BPM-194:Y", "SR-DI-BPM-195:Y", "SR-DI-BPM-196:Y", "SR-DI-BPM-197:Y", "SR-DI-BPM-201:Y", "SR-DI-BPM-202:Y", "SR-DI-BPM-203:Y", "SR-DI-BPM-204:Y", "SR-DI-BPM-205:Y", "SR-DI-BPM-206:Y", "SR-DI-BPM-207:Y", "SR-DI-BPM-208:Y", "SR-DI-BPM-210:Y", "SR-DI-BPM-211:Y", "SR-DI-BPM-212:Y", "SR-DI-BPM-213:Y", "SR-DI-BPM-214:Y", "SR-DI-BPM-215:Y", "SR-DI-BPM-216:Y", "SR-DI-BPM-217:Y", "SR-DI-BPM-221:Y", "SR-DI-BPM-222:Y", "SR-DI-BPM-223:Y", "SR-DI-BPM-224:Y", "SR-DI-BPM-225:Y", "SR-DI-BPM-226:Y", "SR-DI-BPM-227:Y", "SR-DI-BPM-231:Y", "SR-DI-BPM-232:Y", "SR-DI-BPM-233:Y", "SR-DI-BPM-234:Y", "SR-DI-BPM-235:Y", "SR-DI-BPM-236:Y", "SR-DI-BPM-237:Y", "SR-DI-BPM-241:Y", "SR-DI-BPM-242:Y", "SR-DI-BPM-243:Y", "SR-DI-BPM-244:Y", "SR-DI-BPM-245:Y", "SR-DI-BPM-246:Y", "SR-DI-BPM-247:Y"]  # sorted BPMY_174
    w308 = string[] ["SR-DI-BPM-011:X", "SR-DI-BPM-012:X", "SR-DI-BPM-013:X", "SR-DI-BPM-014:X", "SR-DI-BPM-015:X", "SR-DI-BPM-016:X", "SR-DI-BPM-017:X", "SR-DI-BPM-021:X", "SR-DI-BPM-022:X", "SR-DI-BPM-023:X", "SR-DI-BPM-024:X", "SR-DI-BPM-025:X", "SR-DI-BPM-026:X", "SR-DI-BPM-027:X", "SR-DI-BPM-031:X", "SR-DI-BPM-032:X", "SR-DI-BPM-033:X", "SR-DI-BPM-034:X", "SR-DI-BPM-035:X", "SR-DI-BPM-036:X", "SR-DI-BPM-037:X", "SR-DI-BPM-041:X", "SR-DI-BPM-042:X", "SR-DI-BPM-043:X", "SR-DI-BPM-044:X", "SR-DI-BPM-045:X", "SR-DI-BPM-046:X", "SR-DI-BPM-047:X", "SR-DI-BPM-048:X", "SR-DI-BPM-050:X", "SR-DI-BPM-051:X", "SR-DI-BPM-052:X", "SR-DI-BPM-053:X", "SR-DI-BPM-054:X", "SR-DI-BPM-055:X", "SR-DI-BPM-056:X", "SR-DI-BPM-057:X", "SR-DI-BPM-061:X", "SR-DI-BPM-062:X", "SR-DI-BPM-063:X", "SR-DI-BPM-064:X", "SR-DI-BPM-065:X", "SR-DI-BPM-066:X", "SR-DI-BPM-067:X", "SR-DI-BPM-071:X", "SR-DI-BPM-072:X", "SR-DI-BPM-073:X", "SR-DI-BPM-074:X", "SR-DI-BPM-075:X", "SR-DI-BPM-076:X", "SR-DI-BPM-077:X", "SR-DI-BPM-081:X", "SR-DI-BPM-082:X", "SR-DI-BPM-083:X", "SR-DI-BPM-084:X", "SR-DI-BPM-085:X", "SR-DI-BPM-086:X", "SR-DI-BPM-087:X", "SR-DI-BPM-091:X", "SR-DI-BPM-092:X", "SR-DI-BPM-093:X", "SR-DI-BPM-094:X", "SR-DI-BPM-095:X", "SR-DI-BPM-096:X", "SR-DI-BPM-097:X", "SR-DI-BPM-101:X", "SR-DI-BPM-102:X", "SR-DI-BPM-103:X", "SR-DI-BPM-104:X", "SR-DI-BPM-105:X", "SR-DI-BPM-106:X", "SR-DI-BPM-107:X", "SR-DI-BPM-111:X", "SR-DI-BPM-112:X", "SR-DI-BPM-113:X", "SR-DI-BPM-114:X", "SR-DI-BPM-115:X", "SR-DI-BPM-116:X", "SR-DI-BPM-117:X", "SR-DI-BPM-121:X", "SR-DI-BPM-122:X", "SR-DI-BPM-123:X", "SR-DI-BPM-124:X", "SR-DI-BPM-125:X", "SR-DI-BPM-126:X", "SR-DI-BPM-127:X", "SR-DI-BPM-128:X", "SR-DI-BPM-130:X", "SR-DI-BPM-131:X", "SR-DI-BPM-132:X", "SR-DI-BPM-133:X", "SR-DI-BPM-134:X", "SR-DI-BPM-135:X", "SR-DI-BPM-136:X", "SR-DI-BPM-137:X", "SR-DI-BPM-141:X", "SR-DI-BPM-142:X", "SR-DI-BPM-143:X", "SR-DI-BPM-144:X", "SR-DI-BPM-145:X", "SR-DI-BPM-146:X", "SR-DI-BPM-147:X", "SR-DI-BPM-151:X", "SR-DI-BPM-152:X", "SR-DI-BPM-153:X", "SR-DI-BPM-154:X", "SR-DI-BPM-155:X", "SR-DI-BPM-156:X", "SR-DI-BPM-157:X", "SR-DI-BPM-161:X", "SR-DI-BPM-162:X", "SR-DI-BPM-163:X", "SR-DI-BPM-164:X", "SR-DI-BPM-165:X", "SR-DI-BPM-166:X", "SR-DI-BPM-167:X", "SR-DI-BPM-171:X", "SR-DI-BPM-172:X", "SR-DI-BPM-173:X", "SR-DI-BPM-174:X", "SR-DI-BPM-175:X", "SR-DI-BPM-176:X", "SR-DI-BPM-177:X", "SR-DI-BPM-181:X", "SR-DI-BPM-182:X", "SR-DI-BPM-183:X", "SR-DI-BPM-184:X", "SR-DI-BPM-185:X", "SR-DI-BPM-186:X", "SR-DI-BPM-187:X", "SR-DI-BPM-191:X", "SR-DI-BPM-192:X", "SR-DI-BPM-193:X", "SR-DI-BPM-194:X", "SR-DI-BPM-195:X", "SR-DI-BPM-196:X", "SR-DI-BPM-197:X", "SR-DI-BPM-201:X", "SR-DI-BPM-202:X", "SR-DI-BPM-203:X", "SR-DI-BPM-204:X", "SR-DI-BPM-205:X", "SR-DI-BPM-206:X", "SR-DI-BPM-207:X", "SR-DI-BPM-208:X", "SR-DI-BPM-210:X", "SR-DI-BPM-211:X", "SR-DI-BPM-212:X", "SR-DI-BPM-213:X", "SR-DI-BPM-214:X", "SR-DI-BPM-215:X", "SR-DI-BPM-216:X", "SR-DI-BPM-217:X", "SR-DI-BPM-221:X", "SR-DI-BPM-222:X", "SR-DI-BPM-223:X", "SR-DI-BPM-224:X", "SR-DI-BPM-225:X", "SR-DI-BPM-226:X", "SR-DI-BPM-227:X", "SR-DI-BPM-231:X", "SR-DI-BPM-232:X", "SR-DI-BPM-233:X", "SR-DI-BPM-234:X", "SR-DI-BPM-235:X", "SR-DI-BPM-236:X", "SR-DI-BPM-237:X", "SR-DI-BPM-241:X", "SR-DI-BPM-242:X", "SR-DI-BPM-243:X", "SR-DI-BPM-244:X", "SR-DI-BPM-245:X", "SR-DI-BPM-246:X", "SR-DI-BPM-247:X"]  # sorted BPMX_174
    w368 = string[] ["BL-05A:HutchA_Enable", "BL-09A:HutchA_Enable", "BL-21A:HutchA_Enable", "BL-23A:HutchA_Enable", "BL-25A:HutchA_Enable", "BL-41A:HutchA_Enable", "BL-45A:HutchA_Enable"]  # Hutch enable
    w387 = string[] ["CPCI03-adl7452-0:doBank0Ch5", "CPCI05-adl7452-0:doBank0Ch5", "CPCI11-adl7452-0:doBank0Ch5", "CPCI12-adl7452-0:doBank0Ch5", "CPCI13-adl7452-0:doBank0Ch5", "CPCI21-adl7452-0:doBank0Ch5", "CPCI23-adl7452-0:doBank0Ch5"]  # FE enable
    (unwired) 1 ("index")
    w464 = 578.303 ("y")
    w469 = 1.202 ("y")
    # "D:\\LOG運轉紀錄\\2016"
    # "45"
    # "41"
    # "25"
    # "23"
    # "21"
    # "09"
    # "05"
    # "0為"
    # "05\n09\n21\n23\n25\n41\n45"
    # "gapMotorOff"
    n33 = disable-structure shown="Disabled" {
      frame Disabled {
        n34 = call-poly <userlib>:"CaLabGet.vi"("PV Name"="TI-INJ-PROC:getTrig-LI-EGUN") -> ("1rst Value (string)"=w624:string)  [unwired: 8 in, 6 out]
        n35 = Equal?(x="1" ("1rst Value (string)"), y=w624) -> (x = y?=w622:bool)
        n36 = case shown="True" w622 {
          frame False {
          }
          frame True {
            n37 = local read item#-1() -> (→"date (last Gun ON)")
            n38 = local read item#-1() -> (→"time string (last Gun ON)")
          }
        }
      }
      frame Enabled {
      }
    }
    n39 = event shown="[3] \"Refresh Button\": Value Change" {
      selector: _ -> [_ _ _ _ _]
      dyn-events: _ -> [_ _ _ _ _]
      timeout: 233 -> [_ _ _ _ _]
      tunnel: [_ w492 _ _ _] -> w54
      tunnel: [w490 w491 w493 w568 w575] -> w53
      tunnel: w52 -> [w490 w491 w493 _ w575]
      event Timeout {
        n40 = event-data() -> ()  [unwired: 1 in, 3 out]
      }
      event "stop": Value Change {
        n41 = event-data() -> ("NewVal"=w492:bool)  [unwired: 1 in, 3 out]
      }
      event "Open Button": Value Change {
        n42 = event-data() -> ()  [unwired: 1 in, 6 out]
        n43 = Get Date/Time In Seconds() -> (seconds since 1Jan1904=w514:timestamp)
        n44 = Format Date/Time String(time format string (%c)="%Y", seconds (now)=w514, UTC format=FALSE) -> (date/time string=w506:string)
        n45 = Format Date/Time String(time format string (%c)="%d", seconds (now)=w514, UTC format=FALSE) -> (date/time string=w497:string)
        n46 = call "to_be_2_string.vi"("string 2"=w497) -> ("substring 2"=w496:string)  [unwired: 10 in]
        n47 = Format Date/Time String(time format string (%c)="%m", seconds (now)=w514, UTC format=FALSE) -> (date/time string=w502:string)
        n48 = Concatenate Strings("D" ("磁碟位置"), ":\\LOG運轉紀錄\\", w506, "\\", w502, "\\", w496) -> (w494:string)
        n49 = String To Path(string=w494) -> (path=w510:path)
        n50 = call <vilib>:"Check if File or Folder Exists.vi"("path"=w510) -> ("error out"=w512:errorcluster, "file or folder exists?"=w498:bool, "dup path"=w511:path)  [unwired: 8 in]
        n51 = case shown="False" w498 {
          tunnel: w511 -> [w521 w523]
          tunnel: w512 -> [w520 w522]
          tunnel: [w519 w523] -> _
          tunnel: [w518 w522] -> w495
          frame False {
            n52 = Create Folder(path (use dialog)=w521, error in=w520) -> (created path=w519:path, error out=w518:errorcluster)  [unwired: 1 in, 1 out]
          }
          frame True {
          }
        }
        n53 = Concatenate Strings("explorer ", w494) -> (w516:string)
        n54 = call <vilib>:"System Exec.vi"("wait until completion? (T)"=FALSE, "error in (no error)"=w495, "command line"=w516) -> ()  [unwired: 5 in, 4 out]
      }
      event "Refresh Button": Value Change {
        n55 = event-data() -> ()  [unwired: 1 in, 1 out]
        n56 = Multiply(x=3600.0 ("y"), y="last ? Hrs") -> (x*y=w545:dbl)
        n57 = Get Date/Time In Seconds() -> (seconds since 1Jan1904=w533:timestamp)
        n58 = Subtract(x=w533, y=w545) -> (x-y=w534:timestamp)
        n59 = call "TimeToString.vi"("Time Stamp Control"=w533) -> ("result string"=w543:string)
        n60 = call "TimeToString.vi"("Time Stamp Control"=w534) -> ("result string"=w544:string)
        n61 = call <vilib>:"Application Directory.vi"() -> ("Application Directory"=w542:path)
        n62 = Build Path(base path=w542, name or relative path="DSN\\172-18-0-32.dsn") -> (appended path=w540:path)
        n63 = call-poly <vilib>:"DB Tools Open Connection.vi"("connection information"=w540) -> ("error out"=w551:errorcluster, "connection reference"=w552:T2)  [unwired: 7 in]
        n64 = Concatenate Strings("SELECT  float_val , smpl_time\nFROM sample \nwhere  channel_id = 104 and smpl_time between '" ("result string"), w544, "' ::timestamp and '" ("result string"), w543, "' ::timestamp" ("result string")) -> (w567:string)
        n65 = call-poly <vilib>:"DB Tools Execute Query.vi"("error in (no error)"=w551, "SQL query"=w567, "connection reference"=w552) -> ("error out"=w554:errorcluster, "recordset reference"=w553:T3)  [unwired: 5 in]
        n66 = call-poly <vilib>:"DB Tools Fetch Recordset Data.vi"("error in (no error)"=w554, "recordset reference"=w553) -> ("error out"=w556:errorcluster, "recordset data"=w559:variant[][], "recordset reference out"=w555:T3)  [unwired: 3 in]
        n67 = call-poly <vilib>:"DB Tools Free Object.vi"("error in (no error)"=w556, "recordset reference"=w555) -> ("error out"=w558:errorcluster, "connection reference"=w557:T2)  [unwired: 8 in]
        n68 = Variant To Data(type=string[][] [], Variant=w559) -> (data=w561:string[][])  [unwired: 1 in, 1 out]
        n69 = call <vilib>:"DB Tools Close Connection.vi"("error in (no error)"=w558, "connection reference"=w557) -> ("error out"=→"error out 2":errorcluster)  [unwired: 5 in]
        n70 = Transpose 2D Array(2D array=w561) -> (transposed array=w563:string[][])
        n71 = Index Array(array=w563, index (row) #1=0 ("index (row)"), index (row) #2=1 ("index (row)")) -> (element #1=w549:string[], element #2=w547:string[])  [unwired: 2 in]
        n72 = for {
          tunnel: w547 -> [w571] mode=indexing
          tunnel: [w570] -> w548 mode=indexing
          n73 = Scan From String "Scan From String"(format string="%<%Y/%m/%d %p %I:%M:%S>T", input string=w571, initial scan location=u32 0, default 1=timestamp(-73814400 s since 1904-01-01)) -> (output 1=w574:timestamp)  [unwired: 1 in, 3 out]
          n74 = To Double Precision Float(number=w574) -> (double precision float=w570:dbl)
        }
        n75 = Fract/Exp String To Number(string=w549) -> (number=w532:dbl[])  [unwired: 3 in, 1 out]
        n76 = Bundle(w548, w532) -> (w568:cluster{dbl[], dbl[]})  [unwired: 1 in]
        n77 = Array Max & Min(array=w532) -> (max value=w524:dbl, min value=w525:dbl)  [unwired: 2 out]
        n78 = Multiply(x=w524, y=1.01) -> (x*y=w530:dbl)
        n79 = Multiply(x=w525, y=0.99) -> (x*y=w528:dbl)
        n80 = Round Toward +Infinity(x=w530) -> (ceil(x): smallest int >= x=w526:dbl)
        n81 = Round Toward -Infinity(1:w528) -> (0:w527:dbl)
        n82 = To Double Precision Float(number=w533) -> (double precision float=w536:dbl)
        n83 = To Double Precision Float(number=w534) -> (double precision float=w537:dbl)
        n84 = control-ref of="BeamCurrent History"() -> (w535:refnum<vi>)
        n85 = property on="Property Node" class="XYGraph (strict)"(reference=w535, "XScale.Maximum"=w536, "XScale.Minimum"=w537, "YScale.Maximum"=w526, "YScale.Minimum"=w527) -> ()  [unwired: 1 in, 2 out]
      }
      event "Save Button": Value Change {
        n86 = event-data() -> ()  [unwired: 1 in, 1 out]
        n87 = Get Date/Time In Seconds() -> (seconds since 1Jan1904=w578:timestamp)
        n88 = Format Date/Time String(time format string (%c)="%Y", seconds (now)=w578, UTC format=FALSE) -> (date/time string=w597:string)
        n89 = Format Date/Time String(time format string (%c)="%d", seconds (now)=w578, UTC format=FALSE) -> (date/time string=w606:string)
        n90 = call "to_be_2_string.vi"("string 2"=w606) -> ("substring 2"=w607:string)  [unwired: 10 in]
        n91 = Format Date/Time String(time format string (%c)="%m", seconds (now)=w578, UTC format=FALSE) -> (date/time string=w601:string)
        n92 = Format Date/Time String(time format string (%c)="%Y%m%d%H%M%S", seconds (now)=w578) -> (date/time string=w585:string)  [unwired: 1 in]
        n93 = Concatenate Strings("D" ("磁碟位置"), ":\\LOG運轉紀錄\\", w597, "\\", w601, "\\", w607) -> (w590:string)
        n94 = String To Path(string=w590) -> (path=w593:path)
        n95 = call <vilib>:"Check if File or Folder Exists.vi"("path"=w593) -> ("error out"=w591:errorcluster, "file or folder exists?"=w605:bool, "dup path"=w592:path)  [unwired: 8 in]
        n96 = invoke on="Cluster" class="Clust (strict)" method="Get Image"() -> ("image data"=w576:T5)  [unwired: 6 in, 5 out]
        n97 = case shown="False" w605 {
          tunnel: w592 -> [w611 w613]
          tunnel: w591 -> [w610 w612]
          tunnel: [w609 w613] -> w577
          tunnel: [w608 w612] -> _
          frame False {
            n98 = Create Folder(path (use dialog)=w611, error in=w610) -> (created path=w609:path, error out=w608:errorcluster)  [unwired: 1 in, 1 out]
          }
          frame True {
          }
        }
        n99 = Path To String(path=w577) -> (string=w589:string)
        n100 = Concatenate Strings(w589, "\\" ("string"), w585) -> (w579:string)
        n101 = Concatenate Strings(w579, ".jpg" ("file format")) -> (w580:string)
        n102 = String To Path(string=w580) -> (path=w584:path)
        n103 = call <vilib>:"Write JPEG File.vi"("quality (80)"=100, "image data"=w576, "path to JPEG file"=w584) -> ("error out"=→"error out 3":errorcluster)  [unwired: 7 in, 1 out]
      }
    }
    n104 = disable-structure shown="Disabled" {
      frame Disabled {
        n105 = Bundle By Name(cluster=T4 {"SR Fill Pattern"=array[864 elements], "Beam Current(mA"=301.91562200000004, "Beam Lifetime(min)"=669.1065769463743, "Beamsize X(um)"=55.54579477590784, "Beamsize Y(um)"=33.648665625479325, "Tune X(from BPM)"=0.1399, "Tune Y(from BPM)"=0.14, "Mode"="Top-Up", "NuX(from BBF) "=0.16718639681347974, "NuY(from BBF)"=0.25219386232318686, "IU22-23gap(R)"=11.0, "IU22-05gap(R)"=7.558, "IU22-05M"=TRUE, "IU22A-09gap(R)"=8.075, "IU22A-09M"=TRUE, "IU22B-09gap(R)"=40.001, "IU22B-09M"=FALSE, "IUT22-21gap(R)"=7.0, "IUT22-21M"=TRUE, "IU22-23M"=TRUE, "IU22A-25gap(R)"=8.18, "IU22A-25M"=TRUE, "IU22B-25gap(R)"=40.0, "IU22B-25M"=FALSE, "EPU48A-41gap(R)"=64.99985000000001, "EPU48A-41gM"=TRUE, "EPU48B-41gap(R)"=65.00399999999999, "EPU48B-41gM"=FALSE, "EPU46-45gap(R)"=45.00005, "EPU46-45gM"=TRUE, "EPU48A-41phase(R)"=0.0001, "EPU48B-41phase(R)"=0.00055, "EPU46-45phase(R)"=0.0, "Grid volt.(V)(S)"=33.0, "Gun mode"="MBM", "Mod.3 HV(kV)(S)"=35.800000000000026, "SR"="SR_DMB_2016_1102_1124LOCO.data", "BR"="Booster_JT_2016_1005_1200.data", "Linac"="Linac2016_1005_0935.data", "LTB"="LTB_JT_2016_1005_1200.data", "BTS"="BTS_2016_1116_1020.data", "RF2 remote"=TRUE, "RF2 OP mode"=TRUE, "RF2 phase.(S)"=-56.70000000000001, "RF Freq.(s)"=499654660.62238467, "RF2 gap volt.(S)"=1400.0, "RF3 remote"=TRUE, "RF3 OP mode"=TRUE, "RF3 phase.(S)"=160.0, "RF3 gap volt.(S)"=1400.0, "BBF V"=TRUE, "BBF H"=TRUE, "BR ext. kicker1(kV)"=18.266, "BR ext. kicker2(kV)"=18.26600000000001, "BR ext. sep.1(V)"=318.8444, "BR ext. sep.2(V)"=444.5, "BR inj. sep.(V)"=105.2, "BR inj. kicker(kV)"=16.40000000000001, "SR kicker4(kV)"=8.27, "SR kicker3(kV)"=8.315, "SR kicker2(kV)"=8.325, "SR kicker1(kV)"=8.4, "SR inj. sep.2(V)"=417.0, "SR inj. sep.1(V)"=419.3416, "Bucket Start"=100.0, "Bucket Last"=630.0, "Bucket Step"=10.0, "Orbit ILK(P)"=TRUE, "IU22-05 Hutch Enable"=TRUE, "IU22A-09M Hutch Enable"=TRUE, "IUT22-21M Hutch Enable"=TRUE, "IU22-23M Hutch Enable"=FALSE, "IU22A-25M Hutch Enable"=TRUE, "EPU48A-41M Hutch Enable"=FALSE, "EPU46-45M Hutch Enable"=TRUE, "EPU46-45 FE Enable"=TRUE, "EPU48A-41 FE Enable"=FALSE, "IU22A-25 FE Enable"=TRUE, "IU22-23 FE Enable"=FALSE, "IUT22-21 FE Enable"=TRUE, "IU22A-09 FE Enable"=TRUE, "IU22-05 FE Enable"=TRUE, "EPU48A-41pM"=TRUE, "EPU48B-41pM"=FALSE, "EPU46-45pM"=FALSE, "Gun volt.(V)(S)"=23.5, "Width count"=30.0, "2ns step"=0.0, "10ps delay"=100.0, "phase shifter"=130.00060000000002, "Taper"=-1.0899999999999999, "05XBPMX 1"=115.877, "09XBPMX 1"=471.421, "21XBPMX 1"=612.331, "23XBPMX 1"=-46.736000000000004, "25XBPMX 1"=462.29900000000004, "41XBPMX 1"=364.139, "45XBPMX 1"=-164.196, "05XBPMY 1"=-62.875, "09XBPMY 1"=-23.034, "21XBPMY 1"=-27.449, "23XBPMY 1"=-89.72200000000001, "25XBPMY 1"=459.291, "41XBPMY 1"=-111.624, "45XBPMY 1"=-57.689, "FOFB H"="On", "FOFB V"="On", "time string"="21:36:25", "date"="2016/11/21", "date (last kicker ON)"="wait to fire", "time string (last kicker ON)"="", "BPMX Graph"={[1, 2, 3, 4, 5, 6, 7, 8, 9, 10, 11, 12, 13, 14, 15, 16, 17, 18, 19, 20, 21, 22, 23, 24, 25, 26, 27, 28, 29, 30, 31, 32, 33, 34, 35, 36, 37, 38, 39, 40, 41, 42, 43, 44, 45, 46, 47, 48, 49, 50, 51, 52, 53, 54, 55, 56, 57, 58, 59, 60, 61, 62, 63, 64, 65, 66, 67, 68, 69, 70, 71, 72, 73, 74, 75, 76, 77, 78, 79, 80, 81, 82, 83, 84, 85, 86, 87, 88, 89, 90, 91, 92, 93, 94, 95, 96, 97, 98, 99, 100, 101, 102, 103, 104, 105, 106, 107, 108, 109, 110, 111, 112, 113, 114, 115, 116, 117, 118, 119, 120, 121, 122, 123, 124, 125, 126, 127, 128, 129, 130, 131, 132, 133, 134, 135, 136, 137, 138, 139, 140, 141, 142, 143, 144, 145, 146, 147, 148, 149, 150, 151, 152, 153, 154, 155, 156, 157, 158, 159, 160, 161, 162, 163, 164, 165, 166, 167, 168, 169, 170, 171, 172, 173, 174], "1rst Value (number)"=[-31.198, -3.303, -73.172, -2.032, 86.386, -75.851, 71.519, -46.03, 6.824, -37.804, 68.275, -4.672, -223.404, -16.867, -6.964, -259.448, -62.697, 1.8880000000000001, 75.267, -92.668, 86.714, -30.843, 12.767, -107.398, -44.436, 161.126, 208.922, 211.488, -27.247, 79.489, 826.962, 470.705, -115.522, -41.497, 159.486, -54.261, -0.64, 42.641, -2.466, -143.394, -24.785, 138.912, -65.805, 42.325, 32.891, -7.298, -96.724, -31.725, 98.531, -80.64, 64.163, 94.83, -44.03, -163.192, 50.589, 46.669000000000004, -87.508, 78.479, 31.618000000000002, -17.077, -125.32600000000001, -3.845, 98.34100000000001, -39.679, 50.247, -58.208, 40.297000000000004, -69.857, 42.548, -19.403, -211.0, -9.082, -322.597, -233.847, -140.75, 97.087, -15.869, -29.053, 59.46, -115.316, 70.896, -60.685, 33.715, 12.09, -520.422, -138.423, -302.753, 79.862, 120.014, 122.671, -55.812, 27.084, 39.115, -138.936, 156.631, 53.777, -72.647, -52.588, 16.002, 45.197, -117.489, 121.709, 27.952, -31.609, -113.58500000000001, 45.019, 55.136, -130.553, 138.93200000000002, 35.998, -30.631, -96.529, -7.589, 100.395, -93.919, 40.569, 79.538, -68.044, -134.578, 2.52, 84.539, -59.166000000000004, 42.576, 34.657000000000004, -15.805, -52.158, 18.484, 4.346, -157.404, 182.672, 202.518, -164.868, -53.871, 8.066, -9.738, -55.594, 92.623, -13.785, 11.587, -60.627, -47.704, 65.516, 57.924, 148.347, -201.348, -302.753, 189.117, 72.681, -134.928, 39.791000000000004, 45.938, -49.072, 54.473, 28.991, -20.657, -80.283, -20.264, 106.907, -121.271, 150.281, -2.243, -11.844, -122.82300000000001, 0.973, 114.186, -107.94, 95.485, 40.314, -36.956, -134.537, 16.196, 91.88, -35.505, -0.018000000000000002]}, "BPMY Graph"={[1, 2, 3, 4, 5, 6, 7, 8, 9, 10, 11, 12, 13, 14, 15, 16, 17, 18, 19, 20, 21, 22, 23, 24, 25, 26, 27, 28, 29, 30, 31, 32, 33, 34, 35, 36, 37, 38, 39, 40, 41, 42, 43, 44, 45, 46, 47, 48, 49, 50, 51, 52, 53, 54, 55, 56, 57, 58, 59, 60, 61, 62, 63, 64, 65, 66, 67, 68, 69, 70, 71, 72, 73, 74, 75, 76, 77, 78, 79, 80, 81, 82, 83, 84, 85, 86, 87, 88, 89, 90, 91, 92, 93, 94, 95, 96, 97, 98, 99, 100, 101, 102, 103, 104, 105, 106, 107, 108, 109, 110, 111, 112, 113, 114, 115, 116, 117, 118, 119, 120, 121, 122, 123, 124, 125, 126, 127, 128, 129, 130, 131, 132, 133, 134, 135, 136, 137, 138, 139, 140, 141, 142, 143, 144, 145, 146, 147, 148, 149, 150, 151, 152, 153, 154, 155, 156, 157, 158, 159, 160, 161, 162, 163, 164, 165, 166, 167, 168, 169, 170, 171, 172, 173, 174], "1rst Value (number)"=[-99.743, 2.851, -30.024, 83.777, -46.733000000000004, -39.889, 2.349, -4.944, 17.022000000000002, 9.824, 11.632, 41.188, -13.992, 13.911, -6.211, 53.857, -48.993, -32.789, -6.3740000000000006, -62.867000000000004, -8.332, 72.09400000000001, -75.398, 53.283, 63.008, -2.23, 43.024, 32.073, -246.641, -93.162, 456.41700000000003, 88.299, 58.803000000000004, 1.7590000000000001, 35.664, 6.575, 18.59, -30.439, 11.254, -28.256, -62.707, -4.503, 1.31, -21.571, 34.77, -8.876, 31.237000000000002, 25.402, 2.726, 20.655, -7.845, -1.443, -31.935000000000002, -16.981, 13.022, 17.515, -82.867, 61.285000000000004, -57.573, 110.363, -27.753, 28.322, -9.241, 53.929, -25.816, 24.231, -57.876, -11.578, 32.087, -70.84, 64.43, 9.409, -157.639, -57.0, 39.267, 30.23, 18.993000000000002, -33.97, 26.195, -10.585, -17.617, -18.667, 31.615000000000002, -25.437, 29.564, 13.537, 6.728, 163.38400000000001, 106.51, -70.056, 12.874, -4.125, -10.855, -21.856, 1.947, 8.096, 11.402000000000001, 5.761, 41.929, -8.752, 18.634, 7.553, -40.034, 39.183, -25.067, -32.557, 5.393, -17.564, -1.614, 20.498, -14.818, 10.313, 35.254, -35.886, 58.359, -36.56, -20.354, 7.593, -21.256, -8.001, -16.79, 10.18, -16.327, 20.416, -10.539, 19.944, -6.801, 13.068, -13.644, 3.468, -0.983, -17.6, 6.785, -26.101, -11.52, 61.191, -32.777, 13.536, 4.026, -14.682, 52.057, -53.883, 27.118000000000002, 31.672, 79.62, 17.715, 15.693, 113.157, -57.095, 14.214, -4.787, -11.148, -3.157, -6.251, -0.764, 3.563, 7.3500000000000005, 10.779, 21.129, 11.36, 7.771, -14.787, -13.278, 0.279, -13.516, -62.422000000000004, -13.389000000000001, 80.56400000000001, -108.465, 69.885, 30.116, 21.421, 32.779, -10.527000000000001]}, "Radio Buttons 2"=enum."absolute", "09XBPMX 2"="", "09XBPMY 2"="", "05XBPMY 2"="", "05XBPMX 2"="", "21XBPMY 2"="", "21XBPMX 2"="", "23XBPMY 2"="", "23XBPMX 2"="", "25XBPMY 2"="", "25XBPMX 2"="", "41XBPMY 2"="", "41XBPMX 2"="", "45XBPMX 2"="", "45XBPMY 2"="", "05 mode"="", "09A mode"="", "09B mode"="", "21 mode"="", "23 mode"="", "25A mode"="", "25B mode"="", "41A mode"="", "41B mode"="", "46 mode"="", "BeamCurrent History"={"BPM NO.  1_172"=[3587880327.0, 3587880337.0, 3587880347.0, 3587880357.0, 3587880367.0, 3587880377.0, 3587880388.0, 3587880398.0, 3587880408.0, 3587880417.0, 3587880427.0, 3587880437.0, 3587880447.0, 3587880457.0, 3587880467.0, 3587880477.0, 3587880487.0, 3587880497.0, 3587880507.0, 3587880517.0, 3587880527.0, 3587880537.0, 3587880547.0, 3587880557.0, 3587880567.0, 3587880577.0, 3587880587.0, 3587880597.0, 3587880607.0, 3587880617.0, 3587880627.0, 3587880637.0, 3587880647.0, 3587880657.0, 3587880667.0, 3587880677.0, 3587880687.0, 3587880697.0, 3587880707.0, 3587880717.0, 3587880727.0, 3587880737.0, 3587880747.0, 3587880757.0, 3587880767.0, 3587880777.0, 3587880787.0, 3587880797.0, 3587880807.0, 3587880817.0, 3587880827.0, 3587880837.0, 3587880847.0, 3587880857.0, 3587880867.0, 3587880877.0, 3587880887.0, 3587880897.0, 3587880907.0, 3587880917.0], [279.8706, 279.6878, 279.5138, 279.3326, 279.1537, 278.9744, 280.1668, 279.9874, 279.8097, 279.6281, 279.4484, 279.2734, 279.0933, 279.9395, 280.0027, 279.8235, 279.642, 279.4661, 279.2873, 279.1089, 279.6484, 280.0044, 279.8243, 279.6482, 279.4694, 279.2899, 279.1109, 279.5519, 279.9906, 279.8127, 279.6339, 279.4608, 279.2828, 279.104, 279.6982, 279.9463, 279.7671, 279.5915, 279.4126, 279.2368, 279.0606, 280.1311, 279.9543, 279.7767, 279.6011, 279.4247, 279.2452, 279.0726, 280.2098, 280.0333, 279.8566, 279.6814, 279.5039, 279.3286, 279.1559, 278.9767, 280.1638, 279.9891, 279.8148, 279.6383]}, "SR Beam Current in Last           Hrs"=12.0} ("Cluster")) -> (w487:T4)  [unwired: 1 in]
        n106 = local write "Cluster"(w487) -> ()
      }
      frame Enabled {
      }
    }
    n107 = call-poly <userlib>:"CaLabGet.vi"("PV Names"=string[] ["FE-DI-XBPM-051:signals:sa.X", "FE-DI-XBPM-051:signals:sa.Y", "FE-DI-XBPM-091:SA:SA_X_MONITOR", "FE-DI-XBPM-091:SA:SA_Y_MONITOR", "FE-DI-XBPM-211:SA:SA_X_MONITOR", "FE-DI-XBPM-211:SA:SA_Y_MONITOR", "FE-DI-XBPM-231:SA:SA_X_MONITOR", "FE-DI-XBPM-231:SA:SA_Y_MONITOR", "FE-DI-XBPM-251:SA:SA_X_MONITOR", "FE-DI-XBPM-251:SA:SA_Y_MONITOR", "FE-DI-XBPM-411:SA:SA_X_MONITOR", "FE-DI-XBPM-411:SA:SA_Y_MONITOR", "FE-DI-XBPM-451:SA:SA_X_MONITOR", "FE-DI-XBPM-451:SA:SA_Y_MONITOR", "FE-DI-XBPM-052:signals:sa.X", "FE-DI-XBPM-052:signals:sa.Y", "FE-DI-XBPM-092:SA:SA_X_MONITOR", "FE-DI-XBPM-092:SA:SA_Y_MONITOR", "FE-DI-XBPM-212:SA:SA_X_MONITOR", "FE-DI-XBPM-212:SA:SA_Y_MONITOR", "FE-DI-XBPM-232:SA:SA_X_MONITOR", "FE-DI-XBPM-232:SA:SA_Y_MONITOR", "FE-DI-XBPM-252:SA:SA_X_MONITOR", "FE-DI-XBPM-252:SA:SA_Y_MONITOR", "FE-DI-XBPM-412:SA:SA_X_MONITOR", "FE-DI-XBPM-412:SA:SA_Y_MONITOR", "FE-DI-XBPM-452:SA:SA_X_MONITOR", "FE-DI-XBPM-452:SA:SA_Y_MONITOR"] ("appended array")) -> ("1rst Value (number)"=w335:dbl[])  [unwired: 8 in, 6 out]
    n108 = Multiply(x=w335, y=0.001) -> (x*y=w334:dbl[])
    "Value Array (number) 7" <- w334
    n109 = disable-structure shown="Disabled" {
      frame Disabled {
        n110 = To Long Integer() -> (32bit integer=w664:i32)  [unwired: 1 in]
        n111 = case shown="1" w664 {
          tunnel: ["Decay" "Top-Up"] -> _
          frame 0, Default {
          }
          frame 1 {
          }
        }
      }
      frame Enabled {
      }
    }
    n112 = Index Array(array=w334, index #1=0 ("index"), index #2=1 ("index"), index #3=2 ("index"), index #4=3 ("index"), index #5=4 ("index"), index #6=5 ("index"), index #7=6 ("index"), index #8=7 ("index"), index #9=8 ("index"), index #10=9 ("index"), index #11=10 ("index"), index #12=11 ("index"), index #13=12 ("index"), index #14=13 ("index"), index #15=14 ("index"), index #16=15 ("index"), index #17=16 ("index"), index #18=17 ("index"), index #19=18 ("index"), index #20=19 ("index"), index #21=20 ("index"), index #22=21 ("index"), index #23=22 ("index"), index #24=23 ("index"), index #25=24 ("index"), index #26=25 ("index"), index #27=26 ("index"), index #28=27 ("index")) -> (element #1=w250:dbl, element #2=w243:dbl, element #3=w249:dbl, element #4=w242:dbl, element #5=w248:dbl, element #6=w241:dbl, element #7=w247:dbl, element #8=w240:dbl, element #9=w246:dbl, element #10=w239:dbl, element #11=w245:dbl, element #12=w238:dbl, element #13=w244:dbl, element #14=w237:dbl, element #15=w136:dbl, element #16=w135:dbl, element #17=w134:dbl, element #18=w133:dbl, element #19=w124:dbl, element #20=w123:dbl, element #21=w118:dbl, element #22=w117:dbl, element #23=w116:dbl, element #24=w115:dbl, element #25=w84:dbl, element #26=w83:dbl, element #27=w82:dbl, element #28=w81:dbl)
    n113 = call-poly <userlib>:"CaLabGet.vi"("PV Names"=string[] ["LI-ES-CPS-01:PULSEMODE", "LI-ES-BPS-01:SETU:GRID", "LI-ES-BPS-01:SETU:MBM", "LI-ES-BPS-01:SETU:SBM", "LI-RF-HVP-31:SET:U", "CPCITM-TI-EVRTG:Pulse6DelaySet", "CPCITM-TI-EVRTG:Pulse7DelaySet", "CPCITM-TI-EVRTG:Pulse6WidthSet", "CPCITM-TI-EVRTG:Pulse7WidthSet", "CPCITM-TI-EVRTG:GTX6CtrlGTXPHSet", "CPCITM-TI-EVRTG:GTX7CtrlGTXPHSet", "CPCITM-TI-EVRTG:GTX6DlySet", "CPCITM-TI-EVRTG:GTX7DlySet"]) -> ("1rst Value (string)"=w397:string[], "1rst Value (number)"=w448:dbl[])  [unwired: 8 in, 5 out]
    "Value Array (number) 3" <- w448
    "1rst Value (string) 2" <- w397
    n114 = call-poly <userlib>:"CaLabGet.vi"("PV Names"=string[] ["BR-PS-INJ-SE:setHV", "BR-PS-INJ-KI:setHV", "BR-PS-EXT-K1:setHV", "BR-PS-EXT-K2:setHV", "BR-PS-EXT-SE1:setHV", "BR-PS-EXT-SE2:setHV", "SR-PS-INJ-SE1:setHV", "SR-PS-INJ-SE2:setHV", "SR-PS-INJ-K1:setHV", "SR-PS-INJ-K2:setHV", "SR-PS-INJ-K3:setHV", "SR-PS-INJ-K4:setHV"]) -> ("1rst Value (number)"=w450:dbl[])  [unwired: 8 in, 6 out]
    "Value Array (number) 2" <- w450
    n115 = call-poly <userlib>:"CaLabGet.vi"("PV Names"=string[] ["SR-RF-MSG:setFreq", "SR-RF2-LLRF:local", "SR-RF2-LLRF:getOperationMode", "SR-RF2-LLRF:getGapVoltage", "SR-RF2-LLRF:setGapVoltage", "SR-RF2-LLRF:setStationPhase", "SR-RF3-LLRF:local", "SR-RF3-LLRF:getOperationMode", "SR-RF3-LLRF:getGapVoltage", "SR-RF3-LLRF:setGapVoltage", "SR-RF3-LLRF:setStationPhase"]) -> ("1rst Value (number)"=w423:dbl[])  [unwired: 8 in, 6 out]
    "Value Array (number) 4" <- w423
    n116 = call-poly <userlib>:"CaLabGet.vi"("PV Names"=string[] ["SR-DI-FP:CurrentBuffer"]) -> ("Value Array (number)"=w405:dbl[][])  [unwired: 8 in, 6 out]
    n117 = call-poly <userlib>:"CaLabGet.vi"("PV Names"=string[] ["TI-INJ-PROC:TopupHiLowStart", "SR-DI-DCCT:BeamCurrent", "SR-DI-DCCT:BeamLifetime", "SR-DI-XPC-40:SigmaX", "SR-DI-XPC-40:SigmaY", "SR-DI-TUNE:nux", "SR-DI-TUNE:nuy", "IGPF:TPSX:SRAM:VEC:PEAKFREQ2", "IGPF:TPSY:SRAM:VEC:PEAKFREQ2", "TI-INJ-PROC:setBucketAddressStart", "TI-INJ-PROC:setBucketAddressLast", "TI-INJ-PROC:setBucketAddressStep"]) -> ("1rst Value (number)"=w484:dbl[])  [unwired: 8 in, 6 out]
    "Value Array (number)" <- w484
    n118 = call-poly <userlib>:"CaLabGet.vi"("PV Names"=string[] ["LI:restoreFilename", "LTB:restoreFilename", "BR:restoreFilename", "BTS:restoreFilename", "SR:restoreFilename"]) -> ("1rst Value (string)"=w407:string[])  [unwired: 8 in, 6 out]
    "1rst Value (string)" <- w407
    n119 = Index Array(array=w397, index=0) -> (element=w395:string)
    n120 = Index Array(array=w448, index #1=0 ("index"), index #2=1 ("index"), index #3=2 ("index"), index #4=3 ("index"), index #5=4 ("index"), index #6=5 ("index"), index #7=6 ("index"), index #8=7 ("index"), index #9=8 ("index"), index #10=9 ("index"), index #11=10 ("index"), index #12=11 ("index"), index #13=12 ("index")) -> (element #2=w283:dbl, element #3=w399:dbl, element #4=w398:dbl, element #5=w281:dbl, element #8=w394:dbl, element #9=w393:dbl, element #10=w392:dbl, element #11=w391:dbl, element #12=w390:dbl, element #13=w389:dbl)  [unwired: 3 out]
    "MBM volt.(S)" <- w399
    "SBM volt.(S)" <- w398
    n121 = Index Array(array=w450, index #1=0 ("index"), index #2=1 ("index"), index #3=2 ("index"), index #4=3 ("index"), index #5=4 ("index"), index #6=5 ("index"), index #7=6 ("index"), index #8=7 ("index"), index #9=8 ("index"), index #10=9 ("index"), index #11=10 ("index"), index #12=11 ("index")) -> (element #1=w296:dbl, element #2=w295:dbl, element #3=w294:dbl, element #4=w293:dbl, element #5=w292:dbl, element #6=w291:dbl, element #7=w290:dbl, element #8=w289:dbl, element #9=w288:dbl, element #10=w287:dbl, element #11=w286:dbl, element #12=w285:dbl)
    n122 = Index Array(array=w423, index #1=0 ("index"), index #2=1 ("index"), index #3=2 ("index"), index #4=3 ("index"), index #5=4 ("index"), index #6=5 ("index"), index #7=6 ("index"), index #8=7 ("index"), index #9=8 ("index"), index #10=9 ("index"), index #11=10 ("index")) -> (element #1=w275:dbl, element #2=w420:dbl, element #3=w418:dbl, element #5=w196:dbl, element #6=w197:dbl, element #7=w415:dbl, element #8=w414:dbl, element #10=w271:dbl, element #11=w272:dbl)  [unwired: 2 out]
    n123 = Index Array(array=w405, index (row)=0 ("index")) -> (element=w265:dbl[])  [unwired: 1 in]
    n124 = Index Array(array=w484, index #1=0 ("index"), index #2=1 ("index"), index #3=2 ("index"), index #4=3 ("index"), index #5=4 ("index"), index #6=5 ("index"), index #7=6 ("index"), index #8=7 ("index"), index #9=8 ("index"), index #10=9 ("index"), index #11=10 ("index"), index #12=11 ("index")) -> (element #1=w482:dbl, element #2=w305:dbl, element #3=w304:dbl, element #4=w470:dbl, element #5=w468:dbl, element #6=w467:dbl, element #7=w466:dbl, element #8=w465:dbl, element #9=w463:dbl, element #10=w299:dbl, element #11=w298:dbl, element #12=w297:dbl)
    n125 = call-poly <userlib>:"CaLabGet.vi"("PV Names"=w166) -> ("1rst Value (number)"=w168:dbl[])  [unwired: 8 in, 6 out]
    n126 = Index Array(array=w407, index #1=0 ("index"), index #2=1 ("index"), index #3=2 ("index"), index #4=3 ("index"), index #5=4 ("index")) -> (element #1=w267:string, element #2=w266:string, element #3=w270:string, element #4=w269:string, element #5=w268:string)
    n127 = call-poly <userlib>:"CaLabGet.vi"("PV Names"=w368) -> ("1rst Value (string)"=w376:string[])  [unwired: 8 in, 6 out]
    n128 = To Byte Integer(number=w168) -> (8bit integer=w167:i8[])
    n129 = for {
      tunnel: w167 -> [w617] mode=indexing
      tunnel: [w614] -> w144 mode=indexing
      n130 = Number To Boolean Array(number=w617) -> (Boolean array=w616:bool[])
      n131 = Index Array(array=w616, index=0) -> (element=w614:bool)
    }
    n132 = for {
      tunnel: w376 -> [w633] mode=indexing
      tunnel: [w632] -> w377 mode=indexing
      n133 = case shown="\"Enable\"" w633 {
        tunnel: [FALSE TRUE] -> w632
        frame "Disable", Default {
        }
        frame "Enable" {
        }
      }
    }
    n134 = call-poly <userlib>:"CaLabGet.vi"("PV Names"=w387) -> ("1rst Value (string)"=w379:string[])  [unwired: 8 in, 6 out]
    n135 = call-poly <userlib>:"CaLabGet.vi"("PV Names"=string[] ["SR-ID-IU22-05:getGap", "SR-ID-IU22A-09:getGap", "SR-ID-IU22B-09:getGap", "SR-ID-IUT22-21:getGap", "SR-ID-IU22-23:getGap", "SR-ID-IU22A-25:getGap", "SR-ID-IU22B-25:getGap", "SR-ID-EPU48A-41:getGap", "SR-ID-EPU48A-41:getPhase", "SR-ID-EPU48B-41:getGap", "SR-ID-EPU48B-41:getPhase", "SR-ID-EPU46-45:getGap", "SR-ID-EPU46-45:getPhase", "SR-ID-IUT22-21:getGapTaper", "SR-ID-EPU48PS-41:getGap"]) -> ("1rst Value (number)"=w367:dbl[])  [unwired: 8 in, 6 out]
    "Value Array (number) 6" <- w367
    n136 = for {
      tunnel: w379 -> [w637] mode=indexing
      tunnel: [w636] -> w378 mode=indexing
      n137 = case shown="\"enable\"" w637 {
        tunnel: [FALSE TRUE] -> w636
        frame "disable", Default {
        }
        frame "enable" {
        }
      }
    }
    n138 = call-poly <userlib>:"CaLabGet.vi"("PV Names"=string[] ["SR-ID-IU22-05:gapMotorOff", "SR-ID-IU22A-09:gapMotorOff", "SR-ID-IU22B-09:gapMotorOff", "SR-ID-IUT22-21:gapMotorOff", "SR-ID-IU22-23:gapMotorOff", "SR-ID-IU22A-25:gapMotorOff", "SR-ID-IU22B-25:gapMotorOff", "SR-ID-EPU48A-41:gapMotorOff", "SR-ID-EPU48B-41:gapMotorOff", "SR-ID-EPU46-45:gapMotorOff", "SR-ID-EPU48A-41:phaseMotorOff", "SR-ID-EPU48B-41:phaseMotorOff", "SR-ID-EPU46-45:phaseMotorOff"]) -> ("1rst Value (string)"=w319:string[])  [unwired: 8 in, 6 out]
    n139 = To Long Integer(number=w418) -> (32bit integer=w419:i32)
    n140 = To Long Integer(number=w420) -> (32bit integer=w421:i32)
    n141 = To Long Integer(number=w414) -> (32bit integer=w417:i32)
    n142 = To Long Integer(number=w415) -> (32bit integer=w416:i32)
    n143 = Index Array(array=w367, index #1=0 ("index"), index #2=1 ("index"), index #3=2 ("index"), index #4=3 ("index"), index #5=4 ("index"), index #6=5 ("index"), index #7=6 ("index"), index #8=7 ("index"), index #9=8 ("index"), index #10=9 ("index"), index #11=10 ("index"), index #12=11 ("index"), index #13=12 ("index"), index #14=13 ("index"), index #15=14 ("index")) -> (element #1=w264:dbl, element #2=w263:dbl, element #3=w262:dbl, element #4=w261:dbl, element #5=w260:dbl, element #6=w259:dbl, element #7=w258:dbl, element #8=w257:dbl, element #9=w256:dbl, element #10=w255:dbl, element #11=w254:dbl, element #12=w253:dbl, element #13=w252:dbl, element #14=w195:dbl, element #15=w251:dbl)
    n144 = for {
      tunnel: w319 -> [w629] mode=indexing
      tunnel: [w628] -> w318 mode=indexing
      n145 = case shown="\"1\", Default" w629 {
        tunnel: [FALSE TRUE] -> w628
        frame "1", Default {
        }
        frame "0" {
        }
      }
    }
    n146 = Index Array(array=w144, index #1=0 ("index"), index #2=1 ("index"), index #3=2 ("index"), index #4=3 ("index"), index #5=4 ("index"), index #6=5 ("index"), index #7=6 ("index"), index #8=7 ("index"), index #9=8 ("index"), index #10=9 ("index"), index #11=10 ("index"), index #12=11 ("index"), index #13=12 ("index"), index #14=13 ("index"), index #15=14 ("index"), index #16=15 ("index"), index #17=16 ("index"), index #18=17 ("index"), index #19=18 ("index"), index #20=19 ("index"), index #21=20 ("index")) -> (element #1=w141:bool, element #2=w140:bool, element #3=w139:bool, element #4=w128:bool, element #5=w127:bool, element #6=w126:bool, element #7=w121:bool, element #8=w120:bool, element #9=w119:bool, element #10=w110:bool, element #11=w109:bool, element #12=w108:bool, element #13=w103:bool, element #14=w102:bool, element #15=w101:bool, element #16=w100:bool, element #17=w99:bool, element #18=w98:bool, element #19=w97:bool, element #20=w96:bool, element #21=w95:bool)
    n147 = case shown="1" w421 {
      tunnel: [FALSE TRUE] -> w277
      frame 0, Default {
      }
      frame 1 {
      }
    }
    n148 = case shown="1" w416 {
      tunnel: [FALSE TRUE] -> w274
      frame 0, Default {
      }
      frame 1 {
      }
    }
    n149 = case shown="0" w419 {
      tunnel: [TRUE FALSE] -> w276
      frame 0 {
      }
      frame 1, Default {
      }
    }
    n150 = case shown="0" w417 {
      tunnel: [TRUE FALSE] -> w273
      frame 0 {
      }
      frame 1, Default {
      }
    }
    n151 = To Long Integer(number=w482) -> (32bit integer=w485:i32)
    n152 = Negate(x=w195) -> (-x=w194:dbl)
    n153 = case shown="1" w485 {
      tunnel: ["Decay" "Top-Up"] -> w306
      frame 0, Default {
      }
      frame 1 {
      }
    }
    n154 = Index Array(array=w377, index #1=0 ("index"), index #2=1 ("index"), index #3=2 ("index"), index #4=3 ("index"), index #5=4 ("index"), index #6=5 ("index"), index #7=6 ("index")) -> (element #1=w142:bool, element #2=w138:bool, element #3=w122:bool, element #4=w105:bool, element #5=w104:bool, element #6=w86:bool, element #7=w85:bool)
    n155 = case shown="\"MBM\", Default" w395 {
      tunnel: ["MBM" "SBM"] -> w284
      tunnel: w399 -> [w643 _]
      tunnel: [w643 w648] -> w282
      tunnel: w398 -> [_ w648]
      tunnel: w394 -> [_ w647]
      tunnel: w393 -> [w642 _]
      tunnel: [w642 w647] -> w280
      tunnel: w392 -> [_ w646]
      tunnel: w391 -> [w641 _]
      tunnel: [w641 w646] -> w279
      tunnel: w390 -> [_ w645]
      tunnel: w389 -> [w640 _]
      tunnel: [w640 w645] -> w278
      frame "MBM", Default {
      }
      frame "SBM" {
      }
    }
    n156 = Multiply(x=w470, y=w469) -> (x*y=w303:dbl)
    n157 = Divide(x=w465, y=w464) -> (x/y=w301:dbl)
    n158 = Multiply(x=w468, y=w469) -> (x*y=w302:dbl)
    n159 = Divide(x=w463, y=w464) -> (x/y=w300:dbl)
    n160 = Index Array(array=w378, index #1=0 ("index"), index #2=1 ("index"), index #3=2 ("index"), index #4=3 ("index"), index #5=4 ("index"), index #6=5 ("index"), index #7=6 ("index")) -> (element #1=w143:bool, element #2=w137:bool, element #3=w125:bool, element #4=w107:bool, element #5=w106:bool, element #6=w88:bool, element #7=w87:bool)
    n161 = call "FE_PAB_OpenState.vi"("FE"=w143, "XBPMX 2"=w136, "XBPMY 2"=w135, "Hutch"=w142, "PAB"=w141, "MGV"=w140, "FCV"=w139) -> ("XBPMX 2"=w132:string, "XBPMY 2"=w131:string)  [unwired: 7 in]
    n162 = call "FE_PAB_OpenState.vi"("FE"=w137, "XBPMX 2"=w134, "XBPMY 2"=w133, "Hutch"=w138, "PAB"=w128, "MGV"=w127, "FCV"=w126) -> ("XBPMX 2"=w130:string, "XBPMY 2"=w129:string)  [unwired: 7 in]
    n163 = call-poly <userlib>:"CaLabGet.vi"("PV Name"="TI-INJ-PROC:getTrig-SR-KICKER") -> ("1rst Value (string)"=w402:string)  [unwired: 8 in, 6 out]
    n164 = Index Array(array=w318, index #1=0 ("index"), index #2=1 ("index"), index #3=2 ("index"), index #4=3 ("index"), index #5=4 ("index"), index #6=5 ("index"), index #7=6 ("index"), index #8=7 ("index"), index #9=8 ("index"), index #10=9 ("index"), index #11=10 ("index"), index #12=11 ("index"), index #13=12 ("index")) -> (element #1=w236:bool, element #2=w235:bool, element #3=w234:bool, element #4=w233:bool, element #5=w232:bool, element #6=w231:bool, element #7=w230:bool, element #8=w229:bool, element #9=w228:bool, element #10=w227:bool, element #11=w226:bool, element #12=w225:bool, element #13=w224:bool)
    n165 = call-poly <userlib>:"CaLabGet.vi"("PV Names"=w308) -> ("1rst Value (number)"=w310:dbl[])  [unwired: 8 in, 6 out]
    n166 = call-poly <userlib>:"CaLabGet.vi"("PV Names"=w309) -> ("1rst Value (number)"=w312:dbl[])  [unwired: 8 in, 6 out]
    n167 = call "FE_PAB_OpenState.vi"("FE"=w125, "XBPMX 2"=w124, "XBPMY 2"=w123, "Hutch"=w122, "PAB"=w121, "MGV"=w120, "FCV"=w119) -> ("XBPMX 2"=w114:string, "XBPMY 2"=w113:string)  [unwired: 7 in]
    n168 = call-poly <userlib>:"CaLabGet.vi"("PV Names"=string[] ["SR-DI-FOFB-H:getStatus", "SR-DI-FOFB-V:getStatus", "IGPF:TPSX:FBCTRL", "IGPF:TPSY:FBCTRL", "TPS-SR-022:bpm3:ilk:enabled", "SR-DI-ANGLE-ILK:StatusX", "SR-DI-ANGLE-ILK:StatusY"]) -> ("1rst Value (string)"=w210:string[], "1rst Value (number)"=w211:dbl[])  [unwired: 8 in, 5 out]
    n169 = call "FE_PAB_OpenState.vi"("FE"=w107, "XBPMX 2"=w118, "XBPMY 2"=w117, "Hutch"=w105, "PAB"=w110, "MGV"=w109, "FCV"=w108) -> ("XBPMX 2"=w112:string, "XBPMY 2"=w111:string)  [unwired: 7 in]
    n170 = Multiply(x=w310, y=w311) -> (x*y=w184:dbl[])
    n171 = To Byte Integer(number=w211) -> (8bit integer=w207:i8[])
    n172 = Multiply(x=w312, y=w311) -> (x*y=w187:dbl[])
    n173 = for {
      tunnel: w207 -> [w619] mode=indexing
      tunnel: [w618] -> w217 mode=indexing
      n174 = case shown="0, Default" w619 {
        tunnel: [TRUE FALSE] -> w618
        frame 1 {
        }
        frame 0, Default {
        }
      }
    }
    n175 = Array Max & Min(array=w184) -> (max value=w186:dbl, min value=w185:dbl)  [unwired: 2 out]
    n176 = Array Max & Min(array=w187) -> (max value=w189:dbl, min value=w188:dbl)  [unwired: 2 out]
    n177 = call "FE_PAB_OpenState.vi"("FE"=w106, "XBPMX 2"=w116, "XBPMY 2"=w115, "Hutch"=w104, "PAB"=w103, "MGV"=w102, "FCV"=w101) -> ("XBPMX 2"=w94:string, "XBPMY 2"=w93:string)  [unwired: 7 in]
    n178 = Index Array(array=w210, index #1=0 ("index"), index #2=1 ("index")) -> (element #1=w205:string, element #2=w204:string)
    n179 = property on="BPMX Graph" class="XYGraph (strict)"("YScale.Maximum"=w186, "YScale.Minimum"=w185) -> ()  [unwired: 2 in, 2 out]
    n180 = call "FE_PAB_OpenState.vi"("FE"=w88, "XBPMX 2"=w84, "XBPMY 2"=w83, "Hutch"=w86, "PAB"=w100, "MGV"=w99, "FCV"=w98) -> ("XBPMX 2"=w92:string, "XBPMY 2"=w91:string)  [unwired: 7 in]
    n181 = property on="BPMY Graph" class="XYGraph (strict)"("YScale.Maximum"=w189, "YScale.Minimum"=w188) -> ()  [unwired: 2 in, 2 out]
    n182 = call "FE_PAB_OpenState.vi"("FE"=w87, "XBPMX 2"=w82, "XBPMY 2"=w81, "Hutch"=w85, "PAB"=w97, "MGV"=w96, "FCV"=w95) -> ("XBPMX 2"=w90:string, "XBPMY 2"=w89:string)  [unwired: 7 in]
    n183 = Bundle("Array 4"=w313, w184) -> (w223:cluster{"Array 4":i32[], dbl[]})  [unwired: 1 in]
    n184 = Bundle("Array 4"=w313, w187) -> (w222:cluster{"Array 4":i32[], dbl[]})  [unwired: 1 in]
    n185 = Index Array(array=w217, index #1=2 ("index"), index #2=3 ("index"), index #3=4 ("index"), index #4=5 ("index"), index #5=6 ("index")) -> (element #1=w203:bool, element #2=w202:bool, element #3=w201:bool)  [unwired: 2 out]
    n186 = Equal?(x="1" ("1rst Value (string)"), y=w402) -> (x = y?=w400:bool)
    "x = y?" <- w400
    n187 = case shown="True" TRUE {
      tunnel: w54 -> [_ w489]
      frame False {
      }
      frame True {
        n188 = Quit LabVIEW(quit? (T)=w489) -> ()
      }
    }
    n189 = case shown="False" w400 {
      tunnel: w467 -> [_ w653]
      tunnel: w466 -> [_ w652]
      tunnel: [w651 w653] -> w193
      tunnel: [w650 w652] -> w192
      tunnel: w191 -> [w651 _]
      tunnel: w190 -> [w650 _]
      frame False {
      }
      frame True {
        n190 = local read "NOW date"() -> (→"date kickeron":string)
        n191 = local read "NOW time"() -> (→"time kickeron":string)
      }
    }
    n192 = Wait Until Next ms Multiple(millisecond multiple=u32 1000) -> ()  [unwired: 1 out]
    n193 = local read "date kickeron"() -> (w199:string)
    n194 = local read "time kickeron"() -> (w198:string)
    n195 = Get Date/Time In Seconds() -> (seconds since 1Jan1904=w315:timestamp)
    n196 = call-poly <userlib>:"CaLabGet.vi"("PV Names"=w80) -> ("1rst Value (string)"=w69:string[])  [unwired: 8 in, 6 out]
    n197 = Format Date/Time String(time format string (%c)="%Y/%m/%d", seconds (now)=w315) -> (date/time string=→"NOW date":string)  [unwired: 1 in]
    n198 = Format Date/Time String(time format string (%c)="%Y/%m/%d", seconds (now)=w315) -> (date/time string=w221:string)  [unwired: 1 in]
    n199 = Format Date/Time String(time format string (%c)="%H:%M:%S", seconds (now)=w315) -> (date/time string=w220:string)  [unwired: 1 in]
    "NOW time" <- w220
    n200 = Index Array(array=w69, index #1=0 ("index"), index #2=1 ("index"), index #3=2 ("index"), index #4=3 ("index"), index #5=4 ("index"), index #6=5 ("index"), index #7=6 ("index"), index #8=7 ("index"), index #9=8 ("index"), index #10=9 ("index")) -> (element #1=w68:string, element #2=w67:string, element #3=w66:string, element #4=w65:string, element #5=w64:string, element #6=w63:string, element #7=w62:string, element #8=w61:string, element #9=w60:string, element #10=w59:string)
    n201 = Bundle By Name(cluster=T4 {"SR Fill Pattern"=array[864 elements], "Beam Current(mA"=301.91562200000004, "Beam Lifetime(min)"=669.1065769463743, "Beamsize X(um)"=55.54579477590784, "Beamsize Y(um)"=33.648665625479325, "Tune X(from BPM)"=0.1399, "Tune Y(from BPM)"=0.14, "Mode"="Top-Up", "NuX(from BBF) "=0.16718639681347974, "NuY(from BBF)"=0.25219386232318686, "IU22-23gap(R)"=11.0, "IU22-05gap(R)"=7.558, "IU22-05M"=TRUE, "IU22A-09gap(R)"=8.075, "IU22A-09M"=TRUE, "IU22B-09gap(R)"=40.001, "IU22B-09M"=FALSE, "IUT22-21gap(R)"=7.0, "IUT22-21M"=TRUE, "IU22-23M"=TRUE, "IU22A-25gap(R)"=8.18, "IU22A-25M"=TRUE, "IU22B-25gap(R)"=40.0, "IU22B-25M"=FALSE, "EPU48A-41gap(R)"=64.99985000000001, "EPU48A-41gM"=TRUE, "EPU48B-41gap(R)"=65.00399999999999, "EPU48B-41gM"=FALSE, "EPU46-45gap(R)"=45.00005, "EPU46-45gM"=TRUE, "EPU48A-41phase(R)"=0.0001, "EPU48B-41phase(R)"=0.00055, "EPU46-45phase(R)"=0.0, "Grid volt.(V)(S)"=33.0, "Gun mode"="MBM", "Mod.3 HV(kV)(S)"=35.800000000000026, "SR"="SR_DMB_2016_1102_1124LOCO.data", "BR"="Booster_JT_2016_1005_1200.data", "Linac"="Linac2016_1005_0935.data", "LTB"="LTB_JT_2016_1005_1200.data", "BTS"="BTS_2016_1116_1020.data", "RF2 remote"=TRUE, "RF2 OP mode"=TRUE, "RF2 phase.(S)"=-56.70000000000001, "RF Freq.(s)"=499654660.62238467, "RF2 gap volt.(S)"=1400.0, "RF3 remote"=TRUE, "RF3 OP mode"=TRUE, "RF3 phase.(S)"=160.0, "RF3 gap volt.(S)"=1400.0, "BBF V"=TRUE, "BBF H"=TRUE, "BR ext. kicker1(kV)"=18.266, "BR ext. kicker2(kV)"=18.26600000000001, "BR ext. sep.1(V)"=318.8444, "BR ext. sep.2(V)"=444.5, "BR inj. sep.(V)"=105.2, "BR inj. kicker(kV)"=16.40000000000001, "SR kicker4(kV)"=8.27, "SR kicker3(kV)"=8.315, "SR kicker2(kV)"=8.325, "SR kicker1(kV)"=8.4, "SR inj. sep.2(V)"=417.0, "SR inj. sep.1(V)"=419.3416, "Bucket Start"=100.0, "Bucket Last"=630.0, "Bucket Step"=10.0, "Orbit ILK(P)"=TRUE, "IU22-05 Hutch Enable"=TRUE, "IU22A-09M Hutch Enable"=TRUE, "IUT22-21M Hutch Enable"=TRUE, "IU22-23M Hutch Enable"=FALSE, "IU22A-25M Hutch Enable"=TRUE, "EPU48A-41M Hutch Enable"=FALSE, "EPU46-45M Hutch Enable"=TRUE, "EPU46-45 FE Enable"=TRUE, "EPU48A-41 FE Enable"=FALSE, "IU22A-25 FE Enable"=TRUE, "IU22-23 FE Enable"=FALSE, "IUT22-21 FE Enable"=TRUE, "IU22A-09 FE Enable"=TRUE, "IU22-05 FE Enable"=TRUE, "EPU48A-41pM"=TRUE, "EPU48B-41pM"=FALSE, "EPU46-45pM"=FALSE, "Gun volt.(V)(S)"=23.5, "Width count"=30.0, "2ns step"=0.0, "10ps delay"=100.0, "phase shifter"=130.00060000000002, "Taper"=-1.0899999999999999, "05XBPMX 1"=115.877, "09XBPMX 1"=471.421, "21XBPMX 1"=612.331, "23XBPMX 1"=-46.736000000000004, "25XBPMX 1"=462.29900000000004, "41XBPMX 1"=364.139, "45XBPMX 1"=-164.196, "05XBPMY 1"=-62.875, "09XBPMY 1"=-23.034, "21XBPMY 1"=-27.449, "23XBPMY 1"=-89.72200000000001, "25XBPMY 1"=459.291, "41XBPMY 1"=-111.624, "45XBPMY 1"=-57.689, "FOFB H"="On", "FOFB V"="On", "time string"="21:36:25", "date"="2016/11/21", "date (last kicker ON)"="wait to fire", "time string (last kicker ON)"="", "BPMX Graph"={[1, 2, 3, 4, 5, 6, 7, 8, 9, 10, 11, 12, 13, 14, 15, 16, 17, 18, 19, 20, 21, 22, 23, 24, 25, 26, 27, 28, 29, 30, 31, 32, 33, 34, 35, 36, 37, 38, 39, 40, 41, 42, 43, 44, 45, 46, 47, 48, 49, 50, 51, 52, 53, 54, 55, 56, 57, 58, 59, 60, 61, 62, 63, 64, 65, 66, 67, 68, 69, 70, 71, 72, 73, 74, 75, 76, 77, 78, 79, 80, 81, 82, 83, 84, 85, 86, 87, 88, 89, 90, 91, 92, 93, 94, 95, 96, 97, 98, 99, 100, 101, 102, 103, 104, 105, 106, 107, 108, 109, 110, 111, 112, 113, 114, 115, 116, 117, 118, 119, 120, 121, 122, 123, 124, 125, 126, 127, 128, 129, 130, 131, 132, 133, 134, 135, 136, 137, 138, 139, 140, 141, 142, 143, 144, 145, 146, 147, 148, 149, 150, 151, 152, 153, 154, 155, 156, 157, 158, 159, 160, 161, 162, 163, 164, 165, 166, 167, 168, 169, 170, 171, 172, 173, 174], "1rst Value (number)"=[-31.198, -3.303, -73.172, -2.032, 86.386, -75.851, 71.519, -46.03, 6.824, -37.804, 68.275, -4.672, -223.404, -16.867, -6.964, -259.448, -62.697, 1.8880000000000001, 75.267, -92.668, 86.714, -30.843, 12.767, -107.398, -44.436, 161.126, 208.922, 211.488, -27.247, 79.489, 826.962, 470.705, -115.522, -41.497, 159.486, -54.261, -0.64, 42.641, -2.466, -143.394, -24.785, 138.912, -65.805, 42.325, 32.891, -7.298, -96.724, -31.725, 98.531, -80.64, 64.163, 94.83, -44.03, -163.192, 50.589, 46.669000000000004, -87.508, 78.479, 31.618000000000002, -17.077, -125.32600000000001, -3.845, 98.34100000000001, -39.679, 50.247, -58.208, 40.297000000000004, -69.857, 42.548, -19.403, -211.0, -9.082, -322.597, -233.847, -140.75, 97.087, -15.869, -29.053, 59.46, -115.316, 70.896, -60.685, 33.715, 12.09, -520.422, -138.423, -302.753, 79.862, 120.014, 122.671, -55.812, 27.084, 39.115, -138.936, 156.631, 53.777, -72.647, -52.588, 16.002, 45.197, -117.489, 121.709, 27.952, -31.609, -113.58500000000001, 45.019, 55.136, -130.553, 138.93200000000002, 35.998, -30.631, -96.529, -7.589, 100.395, -93.919, 40.569, 79.538, -68.044, -134.578, 2.52, 84.539, -59.166000000000004, 42.576, 34.657000000000004, -15.805, -52.158, 18.484, 4.346, -157.404, 182.672, 202.518, -164.868, -53.871, 8.066, -9.738, -55.594, 92.623, -13.785, 11.587, -60.627, -47.704, 65.516, 57.924, 148.347, -201.348, -302.753, 189.117, 72.681, -134.928, 39.791000000000004, 45.938, -49.072, 54.473, 28.991, -20.657, -80.283, -20.264, 106.907, -121.271, 150.281, -2.243, -11.844, -122.82300000000001, 0.973, 114.186, -107.94, 95.485, 40.314, -36.956, -134.537, 16.196, 91.88, -35.505, -0.018000000000000002]}, "BPMY Graph"={[1, 2, 3, 4, 5, 6, 7, 8, 9, 10, 11, 12, 13, 14, 15, 16, 17, 18, 19, 20, 21, 22, 23, 24, 25, 26, 27, 28, 29, 30, 31, 32, 33, 34, 35, 36, 37, 38, 39, 40, 41, 42, 43, 44, 45, 46, 47, 48, 49, 50, 51, 52, 53, 54, 55, 56, 57, 58, 59, 60, 61, 62, 63, 64, 65, 66, 67, 68, 69, 70, 71, 72, 73, 74, 75, 76, 77, 78, 79, 80, 81, 82, 83, 84, 85, 86, 87, 88, 89, 90, 91, 92, 93, 94, 95, 96, 97, 98, 99, 100, 101, 102, 103, 104, 105, 106, 107, 108, 109, 110, 111, 112, 113, 114, 115, 116, 117, 118, 119, 120, 121, 122, 123, 124, 125, 126, 127, 128, 129, 130, 131, 132, 133, 134, 135, 136, 137, 138, 139, 140, 141, 142, 143, 144, 145, 146, 147, 148, 149, 150, 151, 152, 153, 154, 155, 156, 157, 158, 159, 160, 161, 162, 163, 164, 165, 166, 167, 168, 169, 170, 171, 172, 173, 174], "1rst Value (number)"=[-99.743, 2.851, -30.024, 83.777, -46.733000000000004, -39.889, 2.349, -4.944, 17.022000000000002, 9.824, 11.632, 41.188, -13.992, 13.911, -6.211, 53.857, -48.993, -32.789, -6.3740000000000006, -62.867000000000004, -8.332, 72.09400000000001, -75.398, 53.283, 63.008, -2.23, 43.024, 32.073, -246.641, -93.162, 456.41700000000003, 88.299, 58.803000000000004, 1.7590000000000001, 35.664, 6.575, 18.59, -30.439, 11.254, -28.256, -62.707, -4.503, 1.31, -21.571, 34.77, -8.876, 31.237000000000002, 25.402, 2.726, 20.655, -7.845, -1.443, -31.935000000000002, -16.981, 13.022, 17.515, -82.867, 61.285000000000004, -57.573, 110.363, -27.753, 28.322, -9.241, 53.929, -25.816, 24.231, -57.876, -11.578, 32.087, -70.84, 64.43, 9.409, -157.639, -57.0, 39.267, 30.23, 18.993000000000002, -33.97, 26.195, -10.585, -17.617, -18.667, 31.615000000000002, -25.437, 29.564, 13.537, 6.728, 163.38400000000001, 106.51, -70.056, 12.874, -4.125, -10.855, -21.856, 1.947, 8.096, 11.402000000000001, 5.761, 41.929, -8.752, 18.634, 7.553, -40.034, 39.183, -25.067, -32.557, 5.393, -17.564, -1.614, 20.498, -14.818, 10.313, 35.254, -35.886, 58.359, -36.56, -20.354, 7.593, -21.256, -8.001, -16.79, 10.18, -16.327, 20.416, -10.539, 19.944, -6.801, 13.068, -13.644, 3.468, -0.983, -17.6, 6.785, -26.101, -11.52, 61.191, -32.777, 13.536, 4.026, -14.682, 52.057, -53.883, 27.118000000000002, 31.672, 79.62, 17.715, 15.693, 113.157, -57.095, 14.214, -4.787, -11.148, -3.157, -6.251, -0.764, 3.563, 7.3500000000000005, 10.779, 21.129, 11.36, 7.771, -14.787, -13.278, 0.279, -13.516, -62.422000000000004, -13.389000000000001, 80.56400000000001, -108.465, 69.885, 30.116, 21.421, 32.779, -10.527000000000001]}, "Radio Buttons 2"=enum."absolute", "09XBPMX 2"="", "09XBPMY 2"="", "05XBPMY 2"="", "05XBPMX 2"="", "21XBPMY 2"="", "21XBPMX 2"="", "23XBPMY 2"="", "23XBPMX 2"="", "25XBPMY 2"="", "25XBPMX 2"="", "41XBPMY 2"="", "41XBPMX 2"="", "45XBPMX 2"="", "45XBPMY 2"="", "05 mode"="", "09A mode"="", "09B mode"="", "21 mode"="", "23 mode"="", "25A mode"="", "25B mode"="", "41A mode"="", "41B mode"="", "46 mode"="", "BeamCurrent History"={"BPM NO.  1_172"=[3587880327.0, 3587880337.0, 3587880347.0, 3587880357.0, 3587880367.0, 3587880377.0, 3587880388.0, 3587880398.0, 3587880408.0, 3587880417.0, 3587880427.0, 3587880437.0, 3587880447.0, 3587880457.0, 3587880467.0, 3587880477.0, 3587880487.0, 3587880497.0, 3587880507.0, 3587880517.0, 3587880527.0, 3587880537.0, 3587880547.0, 3587880557.0, 3587880567.0, 3587880577.0, 3587880587.0, 3587880597.0, 3587880607.0, 3587880617.0, 3587880627.0, 3587880637.0, 3587880647.0, 3587880657.0, 3587880667.0, 3587880677.0, 3587880687.0, 3587880697.0, 3587880707.0, 3587880717.0, 3587880727.0, 3587880737.0, 3587880747.0, 3587880757.0, 3587880767.0, 3587880777.0, 3587880787.0, 3587880797.0, 3587880807.0, 3587880817.0, 3587880827.0, 3587880837.0, 3587880847.0, 3587880857.0, 3587880867.0, 3587880877.0, 3587880887.0, 3587880897.0, 3587880907.0, 3587880917.0], [279.8706, 279.6878, 279.5138, 279.3326, 279.1537, 278.9744, 280.1668, 279.9874, 279.8097, 279.6281, 279.4484, 279.2734, 279.0933, 279.9395, 280.0027, 279.8235, 279.642, 279.4661, 279.2873, 279.1089, 279.6484, 280.0044, 279.8243, 279.6482, 279.4694, 279.2899, 279.1109, 279.5519, 279.9906, 279.8127, 279.6339, 279.4608, 279.2828, 279.104, 279.6982, 279.9463, 279.7671, 279.5915, 279.4126, 279.2368, 279.0606, 280.1311, 279.9543, 279.7767, 279.6011, 279.4247, 279.2452, 279.0726, 280.2098, 280.0333, 279.8566, 279.6814, 279.5039, 279.3286, 279.1559, 278.9767, 280.1638, 279.9891, 279.8148, 279.6383]}, "SR Beam Current in Last           Hrs"=12.0} ("Cluster"), "Tune X(from BPM)"=w193, "Tune Y(from BPM)"=w192, "date (last kicker ON)"=w199, "time string (last kicker ON)"=w198, "date"=w221, "time string"=w220, "Mode"=w306, "Beam Current(mA"=w305, "Beam Lifetime(min)"=w304, "Beamsize X(um)"=w303, "Beamsize Y(um)"=w302, "NuX(from BBF)"=w301, "NuY(from BBF)"=w300, "Bucket Start"=w299, "Bucket Last"=w298, "Bucket Step"=w297, "BR inj. sep.(V)"=w296, "BR inj. kicker(kV)"=w295, "BR ext. kicker1(kV)"=w294, "BR ext. kicker2(kV)"=w293, "BR ext. sep.1(V)"=w292, "BR ext. sep.2(V)"=w291, "SR inj. sep.1(V)"=w290, "SR inj. sep.2(V)"=w289, "SR kicker1(kV)"=w288, "SR kicker2(kV)"=w287, "SR kicker3(kV)"=w286, "SR kicker4(kV)"=w285, "Gun mode"=w284, "Grid volt.(V)(S)"=w283, "Gun volt.(V)(S)"=w282, "Mod.3 HV(kV)(S)"=w281, "Width count"=w280, "2ns step"=w279, "10ps delay"=w278, "RF2 remote"=w277, "RF2 OP mode"=w276, "RF2 phase.(S)"=w197, "RF Freq.(s)"=w275, "RF2 gap volt.(S)"=w196, "RF3 remote"=w274, "RF3 OP mode"=w273, "RF3 phase.(S)"=w272, "RF3 gap volt.(S)"=w271, "BR"=w270, "BTS"=w269, "Linac"=w267, "LTB"=w266, "SR"=w268, "SR Fill Pattern"=w265, "IU22-05 Hutch Enable"=w142, "IU22A-09M Hutch Enable"=w138, "IUT22-21M Hutch Enable"=w122, "IU22-23M Hutch Enable"=w105, "IU22A-25M Hutch Enable"=w104, "EPU48A-41M Hutch Enable"=w86, "EPU46-45M Hutch Enable"=w85, "EPU46-45 FE Enable"=w87, "EPU48A-41 FE Enable"=w88, "IU22A-25 FE Enable"=w106, "IU22-23 FE Enable"=w107, "IUT22-21 FE Enable"=w125, "IU22A-09 FE Enable"=w137, "IU22-05 FE Enable"=w143, "IU22-05gap(R)"=w264, "IU22A-09gap(R)"=w263, "IU22B-09gap(R)"=w262, "IUT22-21gap(R)"=w261, "IU22-23gap(R)"=w260, "IU22A-25gap(R)"=w259, "IU22B-25gap(R)"=w258, "EPU48A-41gap(R)"=w257, "EPU48A-41phase(R)"=w256, "EPU48B-41gap(R)"=w255, "EPU48B-41phase(R)"=w254, "EPU46-45gap(R)"=w253, "EPU46-45phase(R)"=w252, "Taper"=w194, "phase shifter"=w251, "05XBPMX 1"=w250, "09XBPMX 1"=w249, "21XBPMX 1"=w248, "23XBPMX 1"=w247, "25XBPMX 1"=w246, "41XBPMX 1"=w245, "45XBPMX 1"=w244, "05XBPMY 1"=w243, "09XBPMY 1"=w242, "21XBPMY 1"=w241, "23XBPMY 1"=w240, "25XBPMY 1"=w239, "41XBPMY 1"=w238, "45XBPMY 1"=w237, "IU22-05M"=w236, "IU22A-09M"=w235, "IU22B-09M"=w234, "IUT22-21M"=w233, "IU22-23M"=w232, "IU22A-25M"=w231, "IU22B-25M"=w230, "EPU48A-41gM"=w229, "EPU48B-41gM"=w228, "EPU46-45gM"=w227, "EPU48A-41pM"=w226, "EPU48B-41pM"=w225, "EPU46-45pM"=w224, "BPMX Graph"=w223, "BPMY Graph"=w222, "Radio Buttons 2"=enum32{"absolute", "different with"}."absolute", "FOFB H"=w205, "FOFB V"=w204, "BBF H"=w203, "BBF V"=w202, "Orbit ILK(P)"=w201, "05XBPMX 2"=w132, "05XBPMY 2"=w131, "09XBPMX 2"=w130, "09XBPMY 2"=w129, "21XBPMX 2"=w114, "21XBPMY 2"=w113, "23XBPMX 2"=w112, "23XBPMY 2"=w111, "25XBPMX 2"=w94, "25XBPMY 2"=w93, "41XBPMX 2"=w92, "41XBPMY 2"=w91, "45XBPMX 2"=w90, "45XBPMY 2"=w89, "05 mode"=w68, "09A mode"=w67, "09B mode"=w66, "21 mode"=w65, "23 mode"=w64, "25A mode"=w63, "25B mode"=w62, "41A mode"=w61, "41B mode"=w60, "46 mode"=w59, "BeamCurrent History"=w53) -> (→"Cluster":T4)
  }
  n202 = local write "stop"(FALSE ("stop")) -> ()
